vi "SO2 43i Serial Data Recording & DECADEv4.3.vi"() -> ()   [LabVIEW 2014]
uses:
  <vilib>/Instr/_visa.llb/VISA Set IO Buffer Mask.ctl
  <vilib>/Platform/TimedLoop/XDataNode/timing_clust.ctl
  <vilib>/Platform/TimedLoop/XDataNode/nitl_modes.ctl
  <vilib>/Platform/TimedLoop/XDataNode/wakeup.ctl
  C:/Program Files (x86)/National Instruments/LabVIEW 2014/examples/Data Communication/Network Streams/Simple Network Streams/support/Network Stream Command.ctl
  <vilib>/Utility/error.llb/whitespace.ctl
  <vilib>/Instr/_visa.llb/VISA Configure Serial Port (Instr).vi
  <vilib>/Utility/file.llb/Read From Spreadsheet File (string).vi
  <vilib>/Utility/tcp.llb/UDP Multicast Write-Only Open.vi
  <vilib>/platform/TimedLoop/XDataNode/XDataNode.xnode
  <vilib>/Platform/TimedLoop/XDataNode/XDNodeRunTimeDep.lvlib
  <vilib>/ptbypt/NI_PtbyPt.lvlib
panel:
  out "local\ndummy":bool
  out "cal gas cylinder conc":dbl=500.0 format="%.4g"
  out "calcon save to file":bool
  out "ev8 zero interval":i32=600
  out "Auto Zeroing":bool
  out "Simulate MOCCA Conc":dbl
  out "MOCCA window delay time (sec)":i32=30
  out "MOCCA SO2 Limit":i32=800
  out "SO2 Inflight MOCCA Alarm\n(default = OFF)":bool
  out "ev8 user set time":i32=60
  out "Mean Cal Offset":dbl
  out "Mean Cal\n(default = ON)":bool=TRUE
  out "Default file name":string
  out "Stop File Write":bool
  out "error out 4":errorcluster
  out "V6":bool
  out "V8":bool
  out "V9":bool
  out "error out 2":errorcluster
  in  "MFC_2 SLPM set value":dbl
  out "Value Read 2":string
  out "status 2":bool
  out "MFC 2":dbl[](array[numeric])
  in  "VISA resource name 3":refnum<visa-resource-name>="ASRL4::INSTR"
  in  "timeout (10sec) 3":u32=3000
  out "error out 3":errorcluster
  in  "MFC_3 SLPM set value":dbl=2.0
  out "Value Read 3":string
  out "status":bool
  out "MFC 3":dbl[](array[numeric])
  in  "VISA resource name 2":refnum<visa-resource-name>="ASRL5::INSTR"
  in  "timeout (10sec) 2":u32=3000
  out "Data Array UDP":string[](array[string])
  out "Slope":dbl=1.1
  out "Zero":dbl
  out "Simulate TWA Conc":dbl
  out "8hr_TWA_limit":i32=490
  out "10mins_STEL_limit":i32=800
  out "Simulate STEL Conc":dbl
  out "Simulate\nconc":bool
  out "q_size 2":i32
  out "8hr_so2_avg 2":dbl=1.0
  out "10min_so2_avg":dbl=1.0
  out "q_size":i32
  in  "Clear Display\nErrors":bool
  out "Data Processing":bool
  out "Serial Visa Error":errorcluster
  out "SEPTIC TCP Error Out":errorcluster
  out "TCP packet\nSend to SEPTIC":bool
  out "UDP Time Stamp Offset":i32=1
  out "Data Array TCP":string[](array[string])
  out "UDP packet \nstatus":bool
  out "UDP_Out_Error":errorcluster
  out "FISH TCP Error Out":errorcluster
  out "TCP packet\nSend to FISH":bool
  out "TCP Binary Packet":string
  out "Scan from String Error Counter\nfrom process loop":i32
  out "Read Error Counter\nfrom process loop":i32
  in  "milliseconds to wait":u32=330
  in  "ID":string="µ"
  in  "VISA resource name":refnum<visa-resource-name>="ASRL6::INSTR"
  out "Data In Array":string[](array[string])
  out "UDP_ASCII_Out":string
  out "UDP_Pack_num":u32
  out "Flight Number":string
  in  "dummy":string="00"
  out "Data String":string
  out "Internal packet":string[](array[string])
  out "RAW DATA":string
  in  "stop":bool
  out "Time taken history":u32(graph)
  out "Max Acq Time diff":u32
  out "Acq Time":u32
  out "Number of Send & Read Error\nfrom Acquire Loop":i32
  out "Command In":string
  # "SO2_conc"
  # "PMT_Volt"
  # "Lamp_Volt"
  # "Lamp_Intensity_Hz"
  # "Internal_Temp_degC"
  # "Reaction_Chamber_Temp_degC"
  # "Reaction_Chamber_Press_mmHg"
  # "Sample_Flow_litre_per_minute"
  # "Flag"
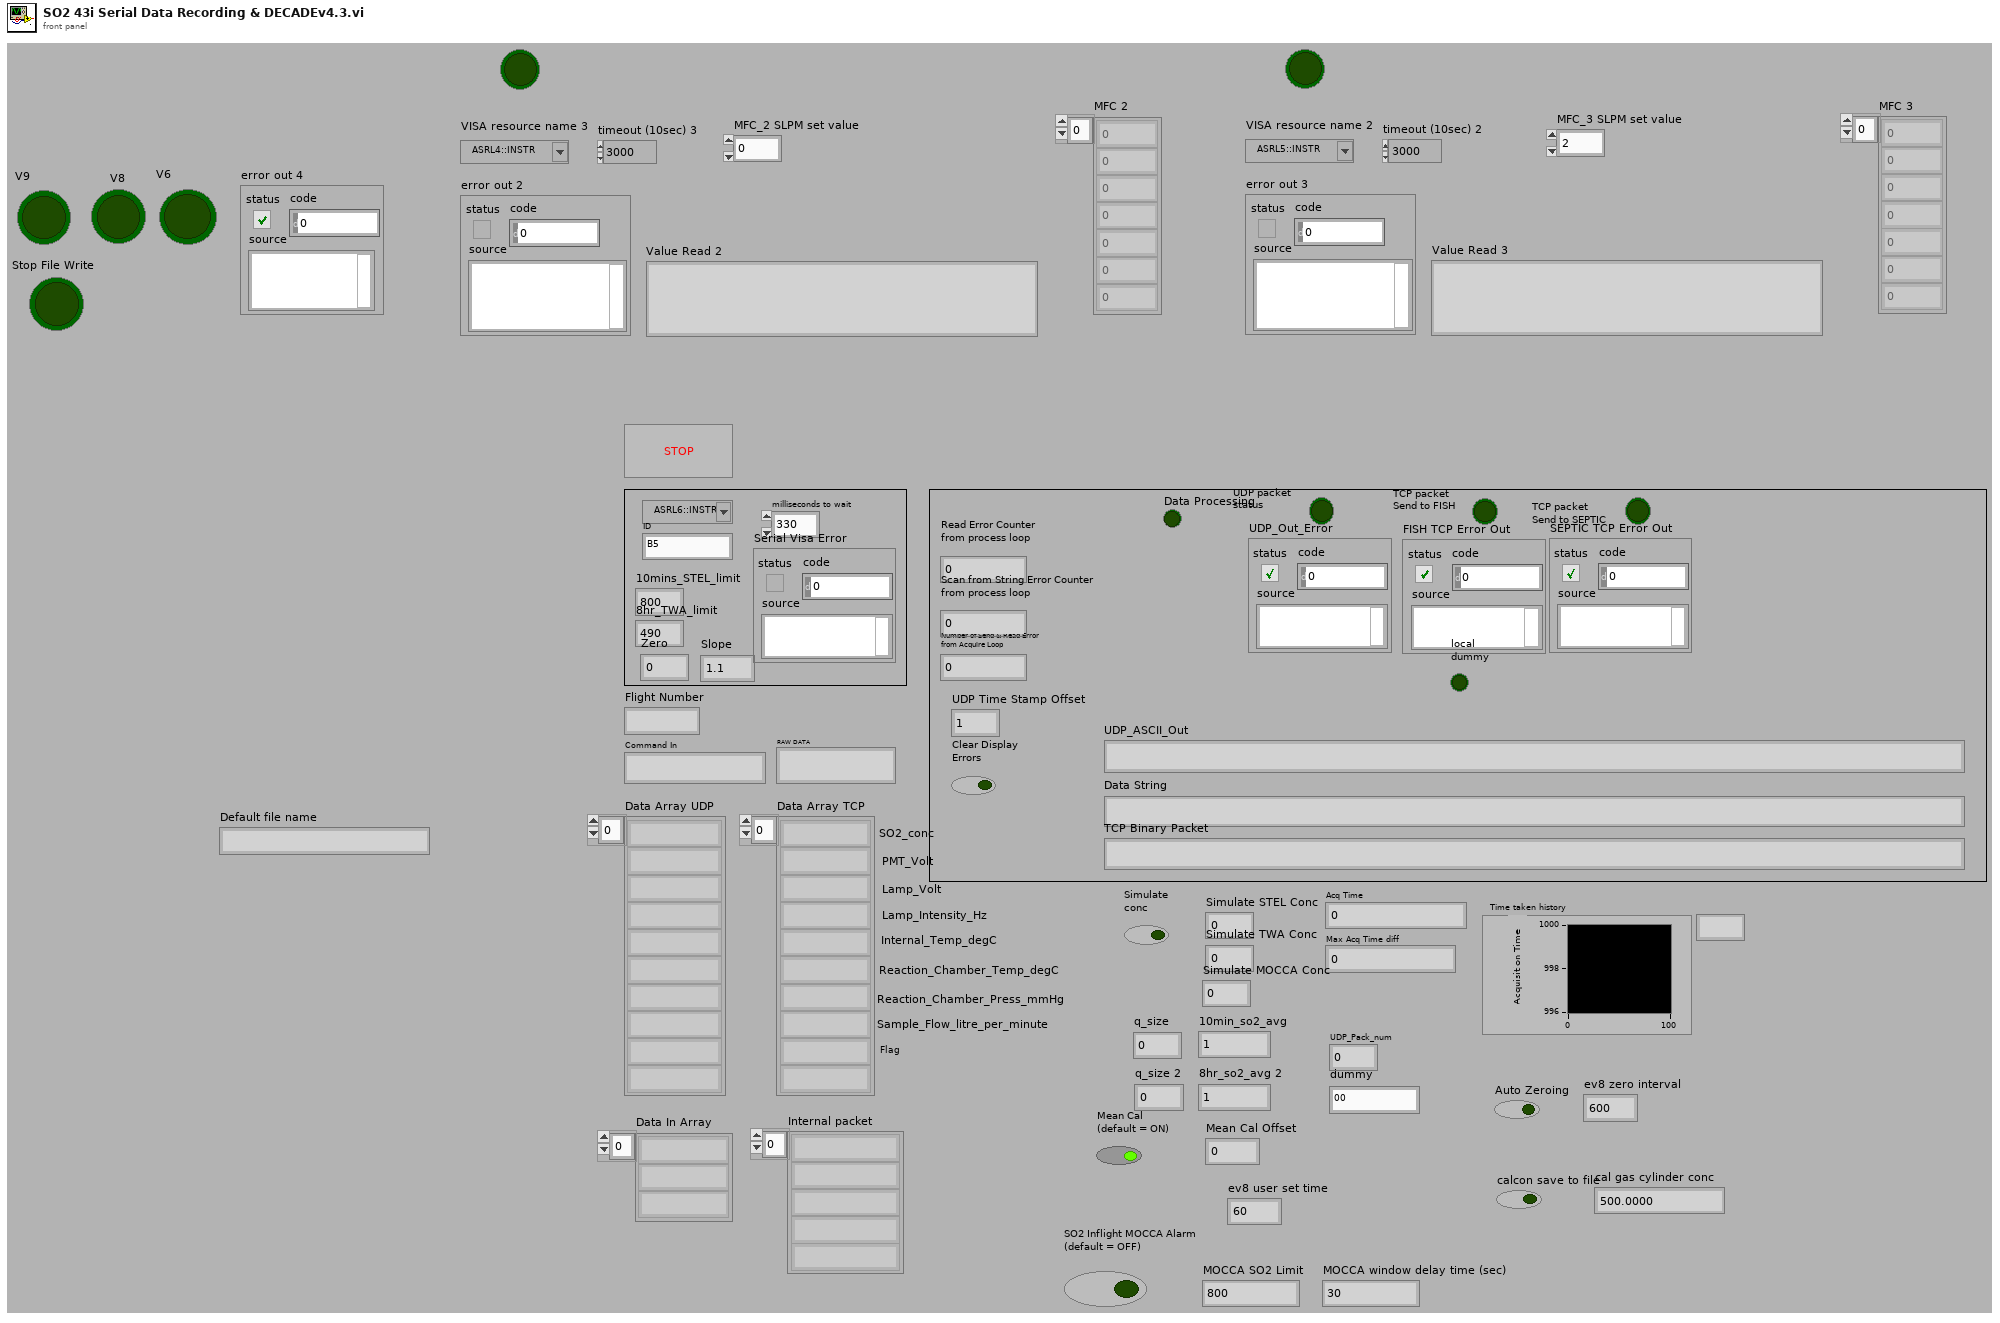
[diagram p1: front panel]
types:
  T1 = typedef "VISA Set IO Buffer Mask.ctl" = u16
  T2 = enum16{"open", "replace", "create", "open or create", "replace or create", "replace or create with confirmation"}
  T3 = typedef "Network Stream Command.ctl" = cluster{"Message":string, "Message Data":variant}
  T4 = typedef "XDNodeRunTimeDep.lvlib/timing_clust.ctl" = cluster{"Expected End [f-1]":u64, "Actual End [f-1]":u64, "Finished Late? [f-1]":bool, "Expected End [i-1]":u64, "Actual End [i-1]":u64, "Finished Late? [i-1]":bool, "Expected Start [i]":u64, "Actual Start [i]":u64, "Expected Start [f]":u64, "Actual Start [f]":u64, "Source Name":string, "Structure Name":string, "Period":i64, "Deadline":i64, "Offset":i64, "Start":i64, "Priority":i32, "Timeout":i32, "Mode":T5, "Wakeup Reason":T6, "Error":errorcluster, "Source Type":string, "Secondary Source Type":string, "Global End Time":u64, "Global Start Time":u64, "Frame Duration":u64, "Iteration Duration":u64, "Assigned CPU":i32, "I/O Scan Engine Mode":u32}
  T5 = typedef "XDNodeRunTimeDep.lvlib/nitl_modes.ctl" = enum32{"No Change", "Process missed periods, maintain original phase", "Discard missed periods, maintain original phase", "Process missed periods, ignore original phase", "Discard missed periods, ignore original phase"}
  T6 = typedef "XDNodeRunTimeDep.lvlib/wakeup.ctl" = enum32{"Normal", "Aborted", "Asynchronous wakeup", "Timing source error", "Timed loop error", "Timeout"}
  T7 = typedef "whitespace.ctl" = u16
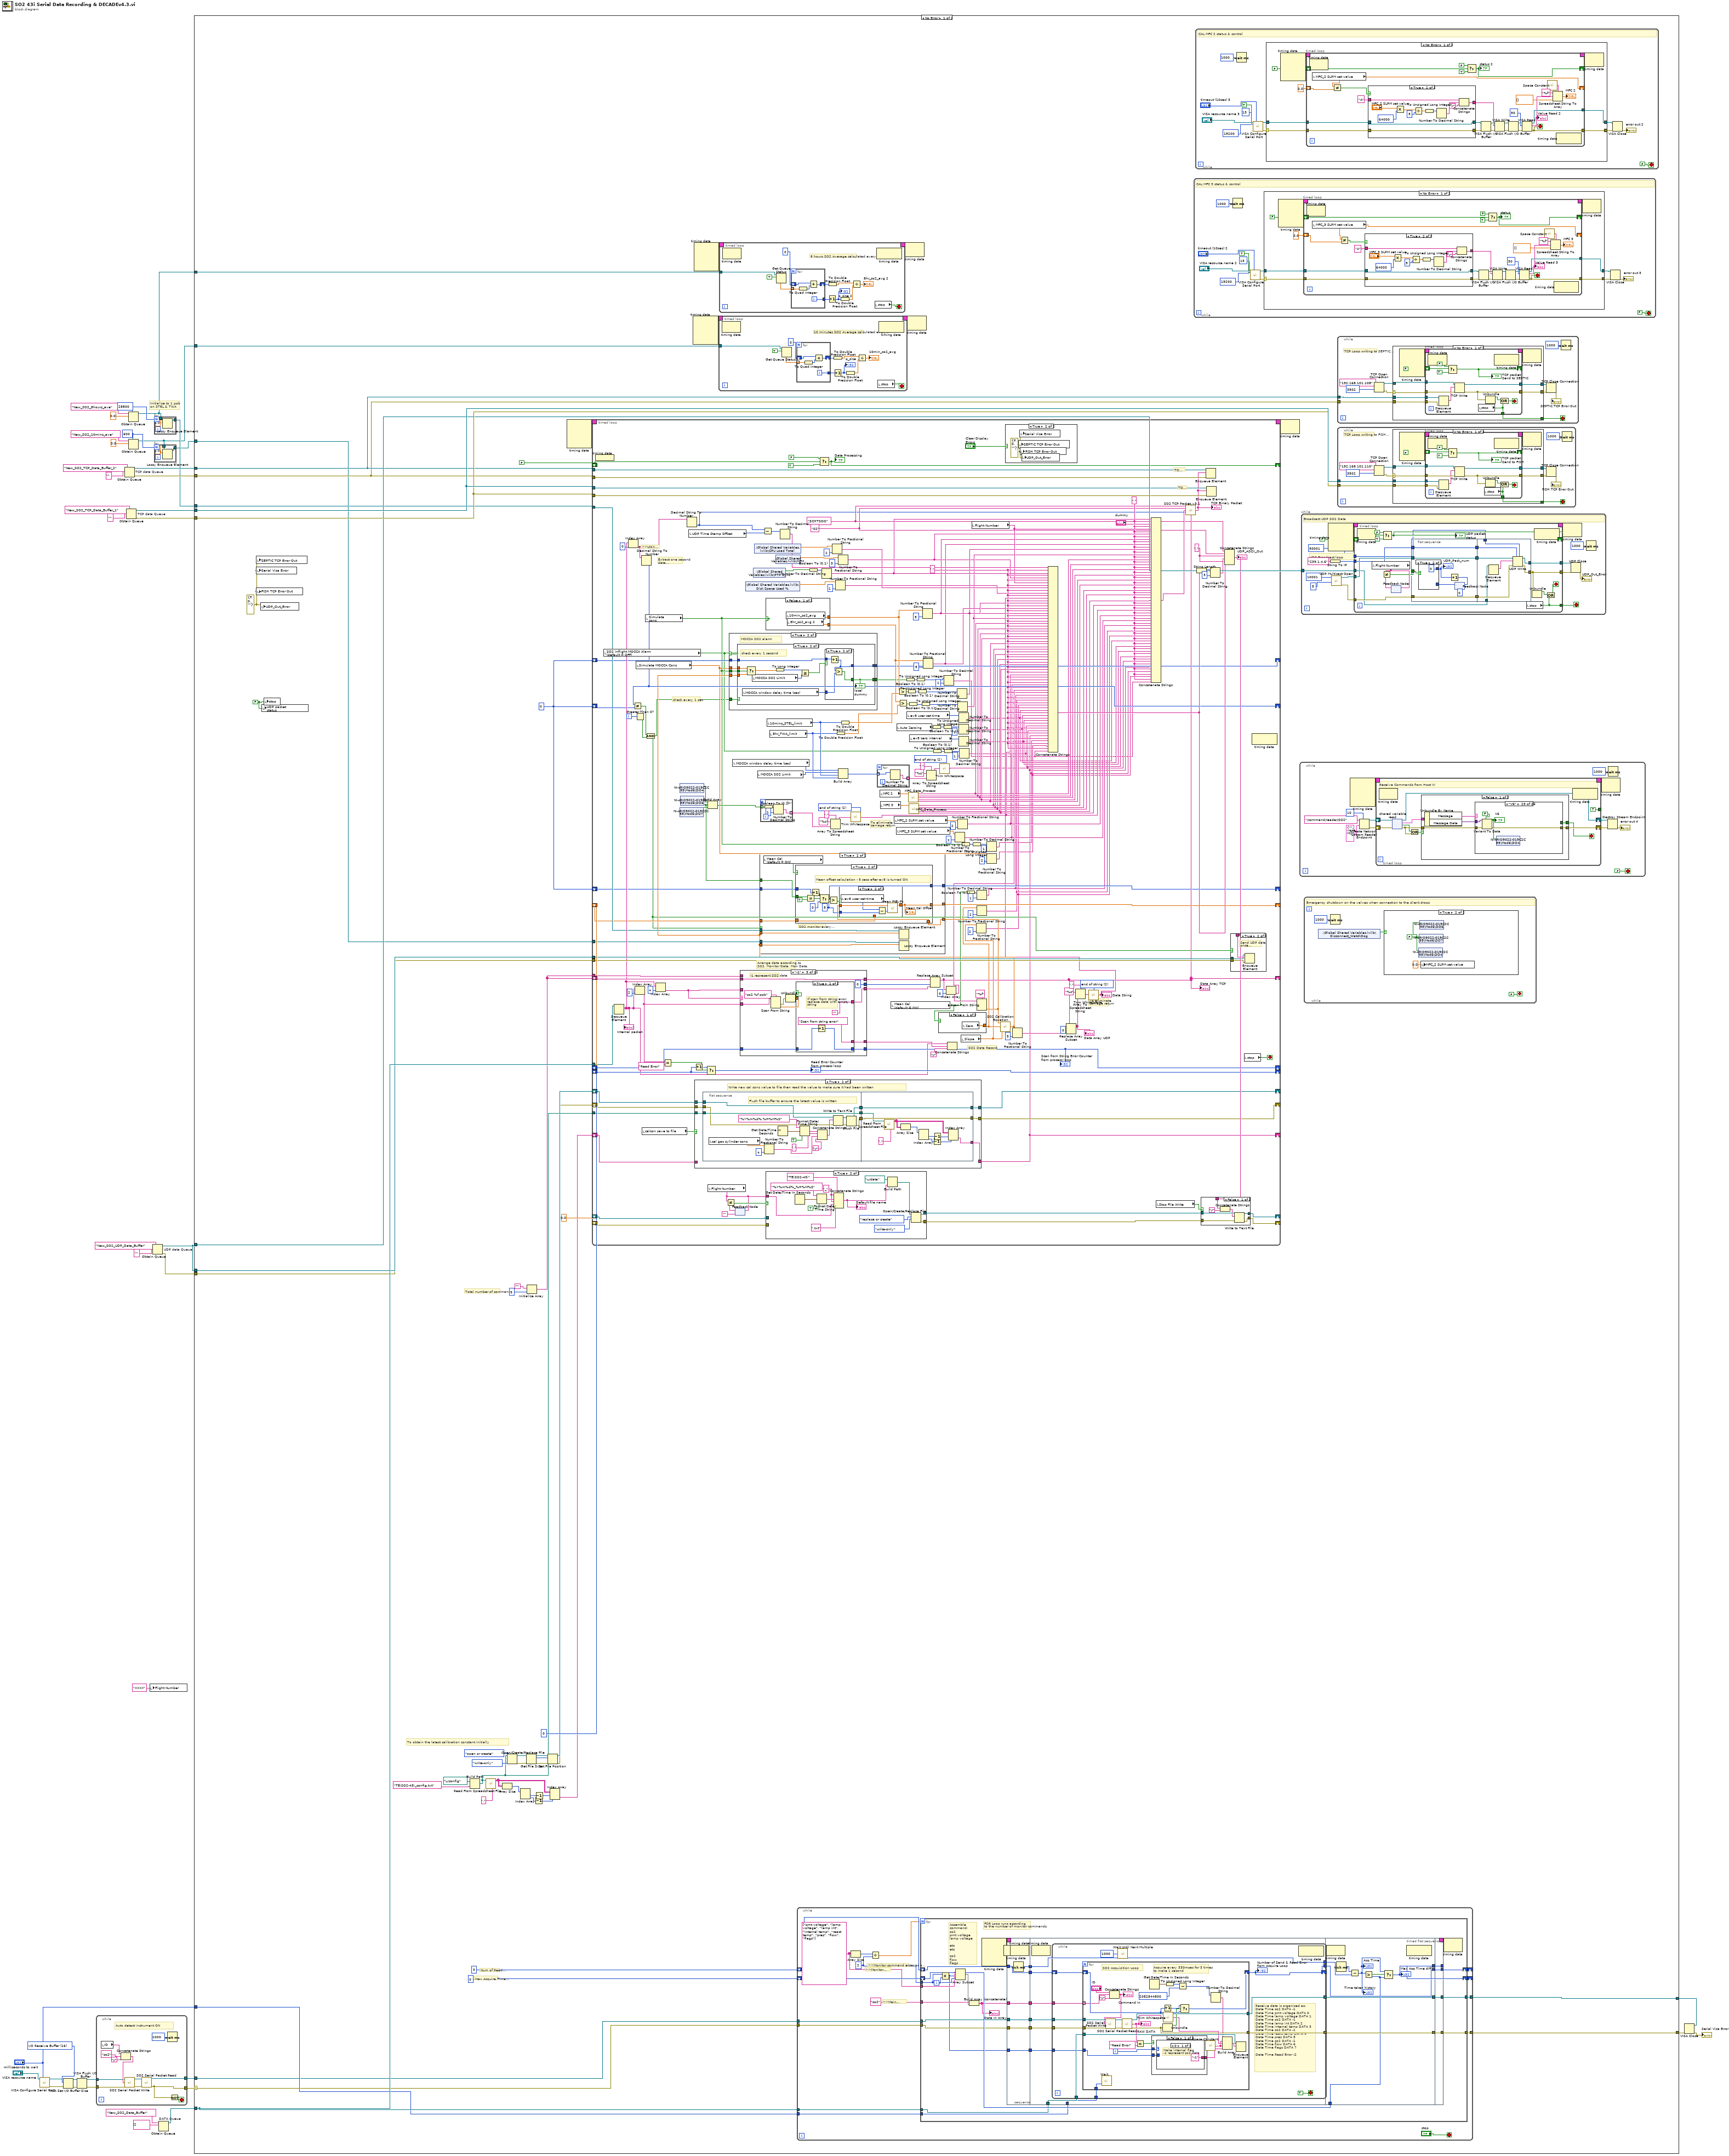
[diagram p0: block diagram]
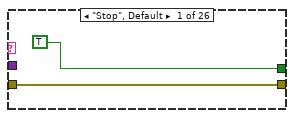
[diagram p3: hidden frame]
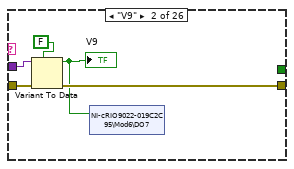
[diagram p4: hidden frame]
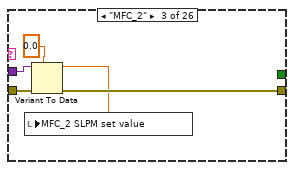
[diagram p5: hidden frame]
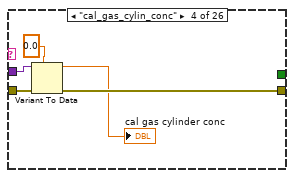
[diagram p6: hidden frame]
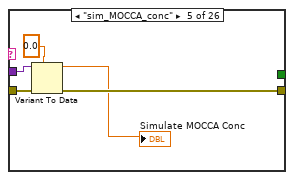
[diagram p7: hidden frame]
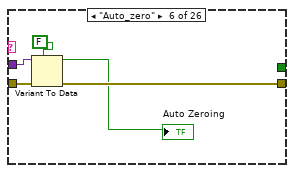
[diagram p8: hidden frame]
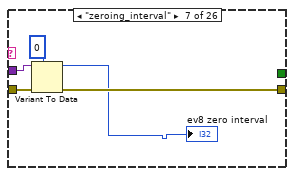
[diagram p9: hidden frame]
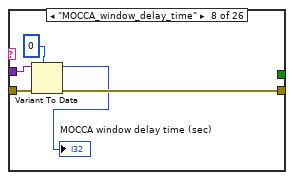
[diagram p10: hidden frame]
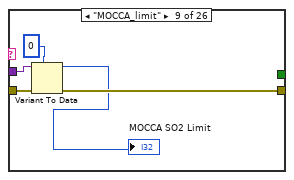
[diagram p11: hidden frame]
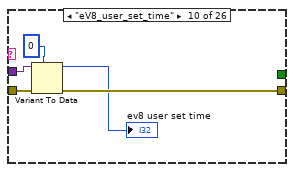
[diagram p12: hidden frame]
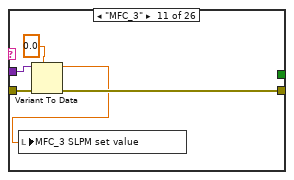
[diagram p13: hidden frame]
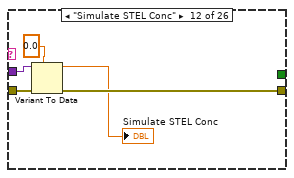
[diagram p14: hidden frame]
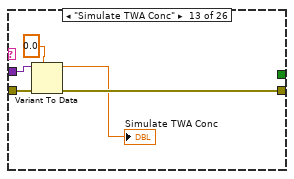
[diagram p15: hidden frame]
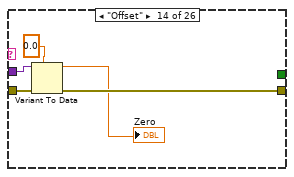
[diagram p16: hidden frame]
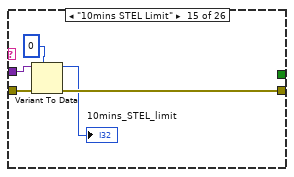
[diagram p17: hidden frame]
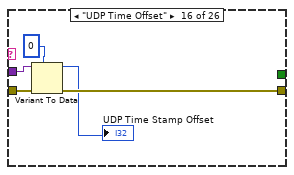
[diagram p18: hidden frame]
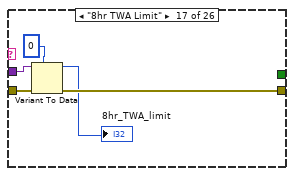
[diagram p19: hidden frame]
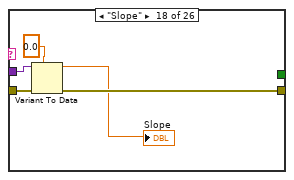
[diagram p20: hidden frame]
diagram:
  w9 = T1 16 items=["I/O Receive Buffer"=16, "I/O Transmit Buffer"=32, "I/O Receive and Transmit Buffer"=48] ("Mask")
  w16 = 28800 ("max queue size (-1, unlimited)")
  w13 = 600 ("max queue size (-1, unlimited)")
  # "Initialise to 1 ppb\non STEL & TWA"
  n1 = call-poly "VISA Configure Serial Port"("VISA resource name"="VISA resource name", "timeout (10sec)"="milliseconds to wait") -> ("VISA resource name out"=w8:refnum<visa-resource-name>, "error out"=w7:errorcluster)  [unwired: 12 in]
  n2 = VISA Set I/O Buffer Size(VISA resource name=w8, mask (16)=w9, error in (no error)=w7) -> (VISA resource name out=w2:refnum<visa-resource-name>, error out=w10:errorcluster)  [unwired: 1 in]
  n3 = VISA Flush I/O Buffer(VISA resource name=w2, error in (no error)=w10) -> (VISA resource name out=w6:refnum<visa-resource-name>, error out=w5:errorcluster)  [unwired: 1 in]
  n4 = while {
    tunnel: w6 -> [w45]
    tunnel: w5 -> [w44]
    tunnel: [w43] -> w4
    tunnel: [w42] -> w3
    stop <- w41 stop-if-true
    # "Auto detect instrument ON"
    n5 = local read "ID"() -> (w46:string)
    n6 = Concatenate Strings(w46, "so2" ("string"), "\r") -> (w49:string)
    n7 = call "SO2 Serial Packet Write.vi"("VISA resource name In"=w45, "Data in"=w49, "error in (no error)"=w44) -> ("VISA resource name Out"=w51:refnum<visa-resource-name>, "error out"=w50:errorcluster)  [unwired: 11 in]
    n8 = call "SO2 Serial Packet Read.vi"("VISA resource In"=w51, "error in"=w50) -> ("VISA resource Out"=w42:refnum<visa-resource-name>, "error out"=w43:errorcluster)  [unwired: 11 in, 1 out]
    n9 = Wait (ms)(milliseconds to wait=u32 1000) -> ()  [unwired: 1 out]
    n10 = Not(x=w43) -> (.not. x?=w41:bool)
  }
  n11 = Obtain Queue "TCP data Queue"(name (unnamed)="New_SO2_TCP_Data_Buffer_2", element data type="") -> (queue out=w23:refnum<queue>, error out=w22:errorcluster)  [unwired: 3 in, 1 out]
  n12 = Obtain Queue "TCP data Queue"(name (unnamed)="New_SO2_TCP_Data_Buffer_1", element data type="") -> (queue out=w31:refnum<queue>, error out=w30:errorcluster)  [unwired: 3 in, 1 out]
  n13 = Obtain Queue(max queue size (-1, unlimited)=w16, name (unnamed)="New_SO2_8hours_ave", element data type=0.0 ("index")) -> (queue out=w15:refnum<queue>)  [unwired: 2 in, 2 out]
  n14 = Obtain Queue(max queue size (-1, unlimited)=w13, name (unnamed)="New_SO2_10mins_ave", element data type=0.0 ("index")) -> (queue out=w12:refnum<queue>)  [unwired: 2 in, 2 out]
  n15 = local write "Flight Number"("XXXX" ("Flight Number")) -> ()
  n16 = Obtain Queue "UDP data Queue"(name (unnamed)="New_SO2_UDP_Data_Buffer", element data type="") -> (queue out=w26:refnum<queue>, error out=w27:errorcluster)  [unwired: 3 in, 1 out]
  n17 = for {
    N: w16 -> [_]
    tunnel: w15 -> [w55]
    tunnel: [w54] -> w14
    n18 = Lossy Enqueue Element(queue=w55, element=1.0) -> (queue out=w54:refnum<queue>)  [unwired: 1 in, 3 out]
  }
  n19 = for {
    N: w13 -> [_]
    tunnel: [w58] -> w11
    tunnel: w12 -> [w56]
    n20 = Lossy Enqueue Element(queue=w56, element=1.0) -> (queue out=w58:refnum<queue>)  [unwired: 1 in, 3 out]
  }
  n21 = Obtain Queue "DATA Queue"(name (unnamed)="New_SO2_Data_Buffer", element data type=string[] []) -> (queue out=w38:refnum<queue>)  [unwired: 3 in, 2 out]
  n22 = case shown="No Error" w4 {
    selector: w4 -> [w81 w1296]
    tunnel: [w112 w1296] -> w35
    tunnel: [w111 w1295] -> w36
    tunnel: w38 -> [w108 _]
    tunnel: w3 -> [w82 w1295]
    tunnel: w31 -> [w100 _]
    tunnel: w30 -> [w99 _]
    tunnel: w26 -> [w98 _]
    tunnel: w27 -> [w97 _]
    tunnel: w26 -> [w96 _]
    tunnel: w23 -> [w95 _]
    tunnel: w22 -> [w94 _]
    tunnel: "milliseconds to wait" -> [w93 _]
    tunnel: w12 -> [w90 _]
    tunnel: w15 -> [w89 _]
    tunnel: w11 -> [w88 _]
    tunnel: w14 -> [w87 _]
    frame No Error {
      w79 = 0
      w91 = errorcluster {"status"=FALSE, "code"=0, "source"=""} ("UDP Error Out")
      w102 = 0
      w101 = FALSE ("stop")
      # "To obtain the latest calibration constant initially"
      # "Max Acquire Time Diff"
      # "Num of Read Error"
      # "Total number of commands"
      n23 = local write "SEPTIC TCP Error Out"(w91) -> ()
      n24 = local write "Serial Visa Error"(w91) -> ()
      n25 = local write "FISH TCP Error Out"(w91) -> ()
      n26 = local write "UDP_Out_Error"(w91) -> ()
      n27 = local write "UDP packet \nstatus"(w101) -> ()
      n28 = local write "stop"(w101) -> ()
      n29 = Build Path(base path=path "u:/config", name or relative path="TEiSO2-43i_config.txt" ("string")) -> (appended path=w61:path)
      n30 = call-poly <vilib>:"Read From Spreadsheet File.vi"("delimiter (\\t)"="," ("delimiter (\\t)"), "file path (dialog if empty)"=w61) -> ("all rows"=w70:string[][])  [unwired: 5 in, 4 out]
      n31 = Array Size(array=w70) -> (size(s)=w71:i32[])
      n32 = Open/Create/Replace File(file path (use dialog)=w61, operation (0:open)=T2."open or create", access (0:read/write)=enum16{"read/write", "read-only", "write-only"}."write-only") -> (refnum out=w63:refnum<file>, error out=w64:errorcluster)  [unwired: 3 in, 1 out]
      n33 = Index Array(array=w71) -> (element #1=w75:i32, element #2=w73:i32)  [unwired: 2 in]
      n34 = Get File Size(file=w63, error in=w64) -> (refnum out=w65:refnum<file>, size (in bytes)=w67:i64, 0:w66:errorcluster)
      n35 = Initialize Array("", 9) -> (w103:string[])
      n36 = Decrement(x=w73) -> (x-1=w72:i32)
      n37 = Decrement(x=w75) -> (x-1=w74:i32)
      n38 = Set File Position(offset (in bytes) (0)=w67, refnum=w65, error in=w66) -> (refnum out=w60:refnum<file>, error out=w59:errorcluster)  [unwired: 1 in]
      n39 = Index Array(array=w70, index (row)=w74, index (col)=w72) -> (element=w69:string)
      n40 = node-c288() -> (w110:T4)  [unwired: 4 in]
      n41 = timed-loop {
        timing: w110 -> [_]
        timing-out: [_] -> w109
        tunnel: w108 -> [w945]
        shift-right: [w877] -> _
        shift-left: w103 -> [w935]
        shift-right: [w926] -> _
        shift-left: w102 -> [w923]
        tunnel: w103 -> [w925]
        shift-right: [w921] -> _
        shift-left: w102 -> [w922]
        tunnel: w100 -> [w919]
        tunnel: w99 -> [w918]
        tunnel: w98 -> [w917]
        tunnel: w97 -> [w916]
        shift-right: [w908] -> _
        shift-left: w79 -> [w911]
        tunnel: w95 -> [w907]
        tunnel: w94 -> [w906]
        shift-right: [w899] -> _
        shift-left: FALSE -> [w902]
        tunnel: w88 -> [w896]
        tunnel: w87 -> [w895]
        shift-right: [w864] -> _
        shift-left: _ -> [w866]
        shift-right: [w863] -> _
        shift-left: _ -> [w865]
        shift-right: [w833] -> _
        shift-left: w79 -> [w835]
        shift-right: [w831] -> _
        shift-left: 0.0 -> [w832]
        shift-right: [w821] -> _
        shift-left: w79 -> [w822]
        tunnel: w61 -> [w798]
        shift-right: [w752] -> _
        shift-left: w69 -> [w797]
        shift-right: [w788] -> _
        shift-left: w60 -> [w789]
        shift-right: [w786] -> _
        shift-left: w59 -> [w787]
        i -> [w909]
        stop <- w943 stop-if-true
        w749 = ","
        (unwired) i16 1 ("width (-)")
        (unwired) T7 2 items=["both", "start of string", "end of string"] ("location (both)")
        w841 = T7 2 items=["both", "start of string", "end of string"] ("location (both)")
        w931 = T7 2 items=["both", "start of string", "end of string"] ("location (both)")
        w791 = ","
        w745 = "02"
        w937 = ","
        w746 = "$CHTSOO"
        # "check every 1 sec"
        # "To eliminate\ncarriage return"
        # "TO SEPTIC"
        # "TO FISH"
        # "Extract one second data\nfor UDP sending"
        # "Arrange data according to\nSO2, Monitor Data, Mon Data,"
        # "To eliminate\ncarriage return"
        # ">>UNIX TIME>>"
        # "SO2 Data Record"
        n42 = node-c288() -> ()  [unwired: 1 in]
        n43 = local read "SO2 Inflight MOCCA Alarm\n(default = OFF)"() -> (w784:bool)
        n44 = Dequeue Element(queue=w945) -> (element=w914:string[])  [unwired: 2 in, 3 out]
        "Internal packet" <- w914
        n45 = Index Array(array=w914, index=0) -> (element=w913:string)
        n46 = Index Array(array=w914, index=2) -> (element=w929:string)
        n47 = Greater Than 0?(x=w909) -> (x > 0?=w912:bool)
        n48 = local read "Simulate MOCCA Conc"() -> (w792:dbl)
        n49 = Decimal String To Number(string=w913) -> (number=w908:i32)  [unwired: 2 in, 1 out]
        n50 = Not Equal?(x=w908, y=w911) -> (x != y?=w910:bool)
        n51 = local read "calcon save to file"() -> (w785:bool)
        n52 = local read "Simulate\nconc"() -> (w794:bool)
        n53 = Compound Arithmetic op=AND(w910, w912) -> (w783:bool)
        n54 = Index Array(array=w914, index=4) -> (element=w898:string)
        n55 = Equal?(x=w929, y="Read Error") -> (x = y?=w927:bool)
        n56 = shared-variable "NI-cRIO9022-019C2C95\\Mod6\\DO7"() -> (w849:bool)  [unwired: 1 in, 1 out]
        n57 = shared-variable "NI-cRIO9022-019C2C95\\Mod6\\DO4"() -> (w850:bool)  [unwired: 1 in, 1 out]
        n58 = shared-variable "NI-cRIO9022-019C2C95\\Mod6\\DO6"() -> (w836:bool)  [unwired: 1 in, 1 out]
        n59 = Decimal String To Number(string=w913) -> (number=w744:i32)  [unwired: 2 in, 1 out]
        n60 = local read "UDP Time Stamp Offset"() -> (w840:i32)
        n61 = Increment(x=w923) -> (x+1=w924:i32)
        n62 = case shown="True" w785 {
          tunnel: w798 -> [_ w957]
          tunnel: [w946 w955] -> w786
          tunnel: w797 -> [w948 _]
          tunnel: [w948 w954] -> w752
          tunnel: w789 -> [w947 w952]
          tunnel: [w947 w950] -> w788
          tunnel: w787 -> [w946 w949]
          frame False {
          }
          frame True {
            # "Write new cal conc value to file then read the value to make sure it had been written"
            n63 = flat-sequence {
              tunnel: w957 -> [w965]
              tunnel: [w960] -> w956
              tunnel: [w965] -> w953
              tunnel: w952 -> [w964]
              tunnel: [w959] -> w951
              tunnel: w949 -> [w963]
              tunnel: w956 -> [w978]
              tunnel: [w978] -> w955
              tunnel: [w977] -> w954
              tunnel: w953 -> [w976]
              tunnel: w951 -> [w975]
              tunnel: [w975] -> w950
              frame #0 {
                # "Flush file buffer to ensure the latest value is written"
                n64 = local read "cal gas cylinder conc"() -> (w958:dbl)
                n65 = Number To Fractional String(number=w958, precision (6)=i16 4) -> (F-format string=w966:string)  [unwired: 2 in]
                n66 = Get Date/Time In Seconds() -> (seconds since 1Jan1904=w973:timestamp)
                n67 = Format Date/Time String(time format string (%c)="%Y%m%d%,%H%M%S", seconds (now)=w973, UTC format=TRUE) -> (date/time string=w970:string)
                n68 = Concatenate Strings(w970, "," ("string"), w966, "\r") -> (w968:string)
                n69 = Write to Text File(file (use dialog)=w964, text=w968, error in=w963) -> (refnum out=w961:refnum<file>, error out=w962:errorcluster)  [unwired: 1 in, 1 out]
                n70 = Flush File(refnum=w961, error in=w962) -> (refnum out=w959:refnum<file>, error out=w960:errorcluster)
              }
              frame #1 {
                n71 = call-poly <vilib>:"Read From Spreadsheet File.vi"("delimiter (\\t)"="," ("delimiter (\\t)"), "file path (dialog if empty)"=w976) -> ("all rows"=w979:string[][])  [unwired: 5 in, 4 out]
                n72 = Array Size(array=w979) -> (size(s)=w980:i32[])
                n73 = Index Array(array=w980) -> (element #1=w984:i32, element #2=w982:i32)  [unwired: 2 in]
                n74 = Decrement(x=w982) -> (x-1=w981:i32)
                n75 = Decrement(x=w984) -> (x-1=w983:i32)
                n76 = Index Array(array=w979, index (row)=w983, index (col)=w981) -> (element=w977:string)
              }
            }
          }
        }
        n77 = Select(t=w924, s=w927, f=w923) -> (s? t:f=w926:i32)
        "Read Error Counter\nfrom process loop" <- w926
        n78 = Build Array(w850, w836, w849) -> (w854:bool[])
        n79 = local read "Flight Number"() -> (w867:string)
        n80 = local read "MOCCA window delay time (sec)"() -> (w803:i32)
        n81 = feedback #1("" ("Flight Number")) -> (w872:string)
        n82 = Not Equal?(x=w867, y=w872) -> (x != y?=w870:bool)
        n83 = feedback-in #1(w867) -> ()
        n84 = case shown="\"-1\"" w898 {
          tunnel: w898 -> [w1094 _ _ w1130 w1151 w1172 w1194 w1216 w1238 w1260 w1282]
          tunnel: w935 -> [w1095 _ w1109 w1131 w1152 w1173 w1195 w1217 w1239 w1261 w1283]
          tunnel: w929 -> [_ _ w1106 w1126 w1147 w1169 w1191 w1213 w1235 w1257 w1279]
          tunnel: [w1095 w1098 w1109 w1131 w1152 w1173 w1195 w1217 w1239 w1261 w1283] -> w882
          tunnel: [w1092 _ 0 ("index") w1128 w1149 w1170 w1192 w1214 w1236 w1258 w1280] -> w881
          tunnel: [_ _ w1105 w1125 w1146 w1168 w1190 w1212 w1234 w1256 w1274] -> w934
          tunnel: w925 -> [_ w1098 _ _ _ _ _ _ _ _ _]
          tunnel: w922 -> [w1090 w1097 w1102 w1122 w1143 w1163 w1186 w1207 w1230 w1251 w1273]
          tunnel: [w1090 w1097 w1101 w1121 w1142 w1162 w1185 w1206 w1229 w1250 w1272] -> w921
          tunnel: ["Internal False Flag Detected" "" w1100 w1120 w1141 w1161 w1184 w1205 w1228 w1249 w1271] -> w920
          frame "False", Default {
            n85 = Decimal String To Number(string=w1094) -> (number=w1091:i32)  [unwired: 2 in, 1 out]
            n86 = Add(x=w1091, y=1) -> (x+y=w1092:i32)
          }
          frame "-2" {
            # "Read Error Detected\nMake all data as a space"
          }
          frame "-1" {
            # "-1 represent SO2 data"
            n87 = Scan From String(format string="so2 %f ppb", input string=w1106) -> (error out=w1104:errorcluster, output 1=w1099:dbl)  [unwired: 3 in, 2 out]
            n88 = Unbundle(w1104) -> ("status"=w1103:bool)  [unwired: 2 out]
            n89 = case shown="True" w1103 {
              tunnel: w1099 -> [w1110 _]
              tunnel: [w1114 ""] -> w1105
              tunnel: w1102 -> [w1113 w1118]
              tunnel: [w1113 w1117] -> w1101
              tunnel: ["" "Scan from string error"] -> w1100
              frame False {
                # "Extract the concentration\nvalue & fixed format"
                n90 = Number To Fractional String(number=w1110, precision (6)=i16 5) -> (F-format string=w1114:string)  [unwired: 2 in]
              }
              frame True {
                # "If scan from string error,\nreplace data with empty\nstring"
                n91 = Increment(x=w1118) -> (x+1=w1117:i32)
              }
            }
          }
          frame "0" {
            # "0 represents pmt voltage -0510 volts"
            n92 = Scan From String(format string="pmt voltage %d", input string=w1126) -> (error out=w1124:errorcluster, output 1=w1119:i32)  [unwired: 3 in, 2 out]
            n93 = Decimal String To Number(string=w1130) -> (number=w1129:i32)  [unwired: 2 in, 1 out]
            n94 = Unbundle(w1124) -> ("status"=w1123:bool)  [unwired: 2 out]
            n95 = case shown="False" w1123 {
              tunnel: w1119 -> [w1135 _]
              tunnel: [w1132 w1136] -> w1125
              tunnel: w1122 -> [w1134 w1139]
              tunnel: [w1134 w1138] -> w1121
              tunnel: ["" "Scan from string error"] -> w1120
              tunnel: [w1132 w1136] -> _
              frame False {
                # "Extract the actual value\n& fixed format"
                n96 = Number To Decimal String(number=w1135) -> (decimal integer string=w1132:string)  [unwired: 1 in]
              }
              frame True {
                w1136 = ""
                # "If scan from string error,\nreplace data with empty\nstring"
                n97 = Increment(x=w1139) -> (x+1=w1138:i32)
              }
            }
            n98 = Increment(x=w1129) -> (x+1=w1128:i32)
          }
          frame "1" {
            # "1 represents lamp voltage; lamp voltage 810 volts"
            n99 = Scan From String(format string="lamp voltage %d", input string=w1147) -> (error out=w1145:errorcluster, output 1=w1140:i32)  [unwired: 3 in, 2 out]
            n100 = Decimal String To Number(string=w1151) -> (number=w1150:i32)  [unwired: 2 in, 1 out]
            n101 = Unbundle(w1145) -> ("status"=w1144:bool)  [unwired: 2 out]
            n102 = case shown="True" w1144 {
              tunnel: w1140 -> [w1156 _]
              tunnel: [w1153 w1157] -> w1146
              tunnel: w1143 -> [w1155 w1160]
              tunnel: [w1155 w1159] -> w1142
              tunnel: ["" "Scan from string error"] -> w1141
              tunnel: [w1153 w1157] -> _
              frame False {
                # "Extract the actual value\n& fixed format"
                n103 = Number To Decimal String(number=w1156) -> (decimal integer string=w1153:string)  [unwired: 1 in]
              }
              frame True {
                w1157 = ""
                # "If scan from string error,\nreplace data with empty\nstring"
                n104 = Increment(x=w1160) -> (x+1=w1159:i32)
              }
            }
            n105 = Increment(x=w1150) -> (x+1=w1149:i32)
          }
          frame "2" {
            # "2 represents lamp intensity; lamp int 35867 Hz"
            n106 = Scan From String(format string="lamp int %d", input string=w1169) -> (error out=w1165:errorcluster, output 1=w1166:i32)  [unwired: 3 in, 2 out]
            n107 = Decimal String To Number(string=w1172) -> (number=w1171:i32)  [unwired: 2 in, 1 out]
            n108 = Unbundle(w1165) -> ("status"=w1164:bool)  [unwired: 2 out]
            n109 = case shown="True" w1164 {
              tunnel: [w1174 w1179] -> w1168
              tunnel: w1166 -> [w1178 _]
              tunnel: w1163 -> [w1177 w1182]
              tunnel: [w1177 w1181] -> w1162
              tunnel: ["" "Scan from string error"] -> w1161
              tunnel: [w1174 w1179] -> _
              frame False {
                # "Extract the actual value\n& fixed format"
                n110 = Number To Fractional String(number=w1178, precision (6)=i16 0) -> (F-format string=w1174:string)  [unwired: 2 in]
              }
              frame True {
                w1179 = ""
                # "If scan from string error,\nreplace data with empty\nstring"
                n111 = Increment(x=w1182) -> (x+1=w1181:i32)
              }
            }
            n112 = Increment(x=w1171) -> (x+1=w1170:i32)
          }
          frame "3" {
            # "3 represents internal temp; internal temp 027.2 deg C, actual 027.2"
            n113 = Scan From String(format string="%[^,], %s %f", input string=w1191) -> (error out=w1188:errorcluster, output 3=w1183:dbl)  [unwired: 7 in, 2 out]
            n114 = Decimal String To Number(string=w1194) -> (number=w1193:i32)  [unwired: 2 in, 1 out]
            n115 = Unbundle(w1188) -> ("status"=w1187:bool)  [unwired: 2 out]
            n116 = case shown="True" w1187 {
              tunnel: [w1196 w1201] -> w1190
              tunnel: w1183 -> [w1200 _]
              tunnel: w1186 -> [w1199 w1204]
              tunnel: [w1199 w1203] -> w1185
              tunnel: ["" "Scan from string error"] -> w1184
              tunnel: [w1196 w1201] -> _
              frame False {
                # "Extract the actual value\n& fixed format"
                n117 = Number To Fractional String(number=w1200, precision (6)=i16 1) -> (F-format string=w1196:string)  [unwired: 2 in]
              }
              frame True {
                w1201 = ""
                # "If scan from string error,\nreplace data with empty\nstring"
                n118 = Increment(x=w1204) -> (x+1=w1203:i32)
              }
            }
            n119 = Increment(x=w1193) -> (x+1=w1192:i32)
          }
          frame "4" {
            # "4 represents react temp; react temp 045.2 deg C"
            n120 = Scan From String(format string="react temp %f deg C", input string=w1213) -> (error out=w1209:errorcluster, output 1=w1210:dbl)  [unwired: 3 in, 2 out]
            n121 = Decimal String To Number(string=w1216) -> (number=w1215:i32)  [unwired: 2 in, 1 out]
            n122 = Unbundle(w1209) -> ("status"=w1208:bool)  [unwired: 2 out]
            n123 = case shown="False" w1208 {
              tunnel: [w1218 w1223] -> w1212
              tunnel: w1210 -> [w1222 _]
              tunnel: w1207 -> [w1221 w1226]
              tunnel: [w1221 w1225] -> w1206
              tunnel: ["" "Scan from string error"] -> w1205
              tunnel: [w1218 w1223] -> _
              frame False {
                # "Extract the actual value\n& fixed format"
                n124 = Number To Fractional String(number=w1222, precision (6)=i16 1) -> (F-format string=w1218:string)  [unwired: 2 in]
              }
              frame True {
                w1223 = ""
                # "If scan from string error,\nreplace data with empty\nstring"
                n125 = Increment(x=w1226) -> (x+1=w1225:i32)
              }
            }
            n126 = Increment(x=w1215) -> (x+1=w1214:i32)
          }
          frame "5" {
            # "5 represents chamber pressure; pres 760.0 mm Hg, actual 753.4"
            n127 = Scan From String(format string="%[^,], %s %f", input string=w1235) -> (error out=w1232:errorcluster, output 3=w1227:dbl)  [unwired: 7 in, 2 out]
            n128 = Decimal String To Number(string=w1238) -> (number=w1237:i32)  [unwired: 2 in, 1 out]
            n129 = Unbundle(w1232) -> ("status"=w1231:bool)  [unwired: 2 out]
            n130 = case shown="False" w1231 {
              tunnel: [w1240 w1245] -> w1234
              tunnel: w1227 -> [w1244 _]
              tunnel: w1230 -> [w1243 w1248]
              tunnel: [w1243 w1247] -> w1229
              tunnel: ["" "Scan from string error"] -> w1228
              tunnel: [w1240 w1245] -> _
              frame False {
                # "Extract the actual value\n& fixed format"
                n131 = Number To Fractional String(number=w1244, precision (6)=i16 1) -> (F-format string=w1240:string)  [unwired: 2 in]
              }
              frame True {
                w1245 = ""
                # "If scan from string error,\nreplace data with empty\nstring"
                n132 = Increment(x=w1248) -> (x+1=w1247:i32)
              }
            }
            n133 = Increment(x=w1237) -> (x+1=w1236:i32)
          }
          frame "6" {
            # "6 represents flow data; flow 0.503 l/m"
            n134 = Scan From String(format string="flow %f l/m", input string=w1257) -> (error out=w1253:errorcluster, output 1=w1254:dbl)  [unwired: 3 in, 2 out]
            n135 = Decimal String To Number(string=w1260) -> (number=w1259:i32)  [unwired: 2 in, 1 out]
            n136 = Unbundle(w1253) -> ("status"=w1252:bool)  [unwired: 2 out]
            n137 = case shown="True" w1252 {
              tunnel: [w1266 ""] -> w1256
              tunnel: w1254 -> [w1265 _]
              tunnel: w1251 -> [w1264 w1269]
              tunnel: [w1264 w1268] -> w1250
              tunnel: ["" "Scan from string error"] -> w1249
              frame False {
                # "Extract the actual value\n& fixed format"
                n138 = Number To Fractional String(number=w1265, precision (6)=i16 3) -> (F-format string=w1266:string)  [unwired: 2 in]
              }
              frame True {
                # "If scan from string error,\nreplace data with empty\nstring"
                n139 = Increment(x=w1269) -> (x+1=w1268:i32)
              }
            }
            n140 = Increment(x=w1259) -> (x+1=w1258:i32)
          }
          frame "7" {
            # "7 represents flags data; flags 1c100000"
            n141 = Scan From String(format string="flags %s", input string=w1279) -> (error out=w1277:errorcluster, output 1=w1275:string)  [unwired: 3 in, 2 out]
            n142 = Decimal String To Number(string=w1282) -> (number=w1281:i32)  [unwired: 2 in, 1 out]
            n143 = Unbundle(w1277) -> ("status"=w1276:bool)  [unwired: 2 out]
            n144 = case shown="False" w1276 {
              tunnel: w1275 -> [w1286 _]
              tunnel: [w1286 ""] -> w1274
              tunnel: w1273 -> [w1285 w1289]
              tunnel: [w1285 w1288] -> w1272
              tunnel: ["" "Scan from string error"] -> w1271
              frame False {
                # "Extract the actual value\n& fixed format"
              }
              frame True {
                # "If scan from string error,\nreplace data with empty\nstring"
                n145 = Increment(x=w1289) -> (x+1=w1288:i32)
              }
            }
            n146 = Increment(x=w1281) -> (x+1=w1280:i32)
          }
        }
        "Scan from String Error Counter\nfrom process loop" <- w921
        n147 = shared-variable ".\\Global Shared Variables.lvlib\\Disk Space Used %"() -> (w843:dbl)  [unwired: 1 in, 1 out]
        n148 = shared-variable ".\\Global Shared Variables.lvlib\\PTP Sync"() -> (w856:bool)  [unwired: 1 in, 1 out]
        n149 = shared-variable ".\\Global Shared Variables.lvlib\\CPU Load Total"() -> (w860:dbl)  [unwired: 1 in, 1 out]
        n150 = local read "MOCCA SO2 Limit"() -> (w802:i32)
        n151 = for {
          tunnel: w854 -> [w1024] mode=indexing
          tunnel: [w1023] -> w851 mode=indexing
          n152 = Boolean To (0,1)(Boolean=w1024) -> (0, 1=w1025:i16)
          n153 = Number To Decimal String(number=w1025, width (-)=i16 1) -> (decimal integer string=w1023:string)
        }
        n154 = Subtract(x=w744, y=w840) -> (x-y=w904:i32)
        n155 = case shown="False" w794 {
          tunnel: [w1017 w1018] -> w891
          tunnel: [w1016 w1019] -> w889
          frame False {
            n156 = local read "10min_so2_avg"() -> (w1017:dbl)
            n157 = local read "8hr_so2_avg 2"() -> (w1016:dbl)
          }
          frame True {
            # "SO2 STEL & TWA simulate"
            n158 = local read "Simulate STEL Conc"() -> (w1018:dbl)
            n159 = local read "Simulate TWA Conc"() -> (w1019:dbl)
          }
        }
        n160 = case shown="True" w870 {
          tunnel: [w1027 w1030] -> w869
          tunnel: [w1026 w1029] -> w868
          tunnel: w866 -> [w1027 _]
          tunnel: w865 -> [w1026 _]
          tunnel: w867 -> [_ w1028]
          frame False {
          }
          frame True {
            w1037 = "_" ("string")
            n161 = Get Date/Time In Seconds() -> (seconds since 1Jan1904=w1038:timestamp)
            n162 = Format Date/Time String(time format string (%c)="%Y%m%d%_%H%M%S", seconds (now)=w1038, UTC format=TRUE) -> (date/time string=w1041:string)
            n163 = Concatenate Strings("TEiSO2-43i" ("string"), w1037, w1041, w1037, w1028, ".txt" ("string")) -> (w1035:string)
            "Default file name" <- w1035
            n164 = Build Path(base path=path "u:/data", name or relative path=w1035) -> (appended path=w1031:path)
            n165 = Open/Create/Replace File(file path (use dialog)=w1031, operation (0:open)=T2."replace or create", access (0:read/write)=enum16{"read/write", "read-only", "write-only"}."write-only") -> (refnum out=w1030:refnum<file>, error out=w1029:errorcluster)  [unwired: 3 in, 1 out]
          }
        }
        n166 = local read "10mins_STEL_limit"() -> (w801:i32)
        n167 = local read "8hr_TWA_limit"() -> (w800:i32)
        n168 = shared-variable ".\\Global Shared Variables.lvlib\\MFM"() -> (w857:dbl)  [unwired: 1 in, 1 out]
        n169 = Number To Decimal String(number=w904) -> (decimal integer string=w903:string)  [unwired: 1 in]
        n170 = Boolean To (0,1)(Boolean=w856) -> (0, 1=w855:i16)
        n171 = Select(t=FALSE, s=w902, f=TRUE) -> (s? t:f=w899:bool)
        "Data Processing" <- w899
        n172 = Number To Decimal String(number=w855) -> (decimal integer string=w782:string)  [unwired: 1 in]
        n173 = Array To Spreadsheet String(delimiter (Tab)=",", array=w851, 3:"%s" ("format string")) -> (spreadsheet string=w842:string)
        n174 = Number To Fractional String(number=w860, precision (6)=i16 2) -> (F-format string=w839:string)  [unwired: 2 in]
        n175 = Number To Fractional String(number=w843, precision (6)=i16 1) -> (F-format string=w838:string)  [unwired: 2 in]
        n176 = To Double Precision Float(number=w800) -> (double precision float=w892:dbl)
        n177 = Number To Fractional String(number=w857, precision (6)=i16 3) -> (F-format string=w774:string)  [unwired: 2 in]
        n178 = Build Array(w803, w802, w801, w800) -> (w799:i32[])
        n179 = To Double Precision Float(number=w801) -> (double precision float=w893:dbl)
        n180 = call <vilib>:"Trim Whitespace.vi"("string"=w842, "location (both)"=w841) -> ("trimmed string"=w763:string)
        n181 = for {
          tunnel: w799 -> [w986] mode=indexing
          tunnel: [w987] -> w805 mode=indexing
          n182 = Number To Decimal String(number=w986) -> (decimal integer string=w987:string)  [unwired: 1 in]
        }
        n183 = local read "MFC 2"() -> (w874:dbl[])
        n184 = local read "MFC 3"() -> (w873:dbl[])
        n185 = local read "Mean Cal\n(default = ON)"() -> (w827:bool)
        n186 = local read "MFC_2 SLPM set value"() -> (w846:dbl)
        n187 = local read "MFC_3 SLPM set value"() -> (w845:dbl)
        n188 = local read "Auto Zeroing"() -> (w813:bool)
        n189 = Greater?(x=w891, y=w893) -> (0:w886:bool)
        n190 = Greater?(x=w889, y=w892) -> (0:w885:bool)
        n191 = Boolean To (0,1)(Boolean=w886) -> (0, 1=w888:i16)
        n192 = local read "ev8 user set time"() -> (w816:i32)
        n193 = Boolean To (0,1)(Boolean=w885) -> (0, 1=w887:i16)
        n194 = call "MFC_Data_Process.vi"("MFC"=w874) -> ("MFC Absolute Pressure"=w773:string, "MFC Temperature"=w772:string, "MFC Volumetric Flow"=w771:string, "MFC Mass Flow"=w770:string, "MFC Set Point"=w769:string)  [unwired: 10 in]
        n195 = call "MFC_Data_Process.vi"("MFC"=w873) -> ("MFC Absolute Pressure"=w768:string, "MFC Temperature"=w767:string, "MFC Volumetric Flow"=w766:string, "MFC Mass Flow"=w765:string, "MFC Set Point"=w764:string)  [unwired: 10 in]
        n196 = local read "ev8 zero interval"() -> (w812:i32)
        n197 = To Unsigned Long Integer(number=w888) -> (unsigned 32bit integer=w884:u32)
        n198 = To Unsigned Long Integer(number=w887) -> (unsigned 32bit integer=w883:u32)
        n199 = Number To Fractional String(number=w891, precision (6)=i16 5) -> (F-format string=w778:string)  [unwired: 2 in]
        n200 = Number To Fractional String(number=w889, precision (6)=i16 5) -> (F-format string=w777:string)  [unwired: 2 in]
        n201 = Array To Spreadsheet String(delimiter (Tab)=",", array=w805, 3:"%s" ("format string")) -> (spreadsheet string=w804:string)
        n202 = Replace Array Subset(array=w882, new element=w934, index=w881) -> (w877:string[])
        "Data Array TCP" <- w877
        n203 = Boolean To (0,1)(Boolean=w813) -> (0, 1=w815:i16)
        n204 = Boolean To (0,1)(Boolean=w784) -> (0, 1=w811:i16)
        n205 = case shown="False" w827 {
          tunnel: [w1020 w1021] -> w824
          frame False {
            n206 = local read "Zero"() -> (w1020:dbl)
          }
          frame True {
            n207 = local read "Mean Cal Offset"() -> (w1021:dbl)
          }
        }
        n208 = call <vilib>:"Trim Whitespace.vi"("string"=w804) -> ("trimmed string"=w753:string)  [unwired: 1 in]
        n209 = To Unsigned Long Integer(number=w815) -> (unsigned 32bit integer=w814:u32)
        n210 = To Unsigned Long Integer(number=w811) -> (unsigned 32bit integer=w810:u32)
        n211 = Index Array(array=w877, index=0) -> (element=w830:string)
        n212 = Concatenate Strings(w914, w920, "\r") -> ()  [unwired: 1 out]
        n213 = Number To Fractional String(number=w845, precision (6)=i16 2) -> (F-format string=w761:string)  [unwired: 2 in]
        n214 = Number To Decimal String(number=w884) -> (decimal integer string=w776:string)  [unwired: 1 in]
        n215 = Number To Decimal String(number=w883) -> (decimal integer string=w775:string)  [unwired: 1 in]
        n216 = Number To Fractional String(number=w846, precision (6)=i16 2) -> (F-format string=w762:string)  [unwired: 2 in]
        n217 = Number To Decimal String(number=w816) -> (decimal integer string=w757:string)  [unwired: 1 in]
        n218 = Number To Decimal String(number=w814, width (-)=i16 1) -> (decimal integer string=w756:string)
        n219 = Number To Decimal String(number=w812) -> (decimal integer string=w755:string)  [unwired: 1 in]
        n220 = Number To Decimal String(number=w810, width (-)=i16 1) -> (decimal integer string=w754:string)
        n221 = Boolean To (0,1)(Boolean=w794) -> (0, 1=w796:i16)
        n222 = local read "Slope"() -> (w823:dbl)
        n223 = Boolean To (0,1)(Boolean=w827) -> (0, 1=w829:i16)
        n224 = local read "Flight Number"() -> (w780:string)
        n225 = To Unsigned Long Integer(number=w796) -> (unsigned 32bit integer=w795:u32)
        n226 = Number To Fractional String(number=w823, precision (6)=i16 2) -> (F-format string=w758:string)  [unwired: 2 in]
        n227 = Number To Decimal String(number=w829, width (-)=i16 1) -> (decimal integer string=w760:string)
        n228 = Number To Fractional String(number=w824, precision (6)=i16 2) -> (F-format string=w759:string)  [unwired: 2 in]
        n229 = Scan From String(format string="%f", input string=w830) -> (output 1=w834:dbl)  [unwired: 3 in, 3 out]
        n230 = Number To Decimal String(number=w795) -> (decimal integer string=w751:string)  [unwired: 1 in]
        n231 = Number To Fractional String(number=w792, precision (6)=i16 2) -> (F-format string=w750:string)  [unwired: 2 in]
        n232 = call "SO2 Calibration Equation.vi"("Input"=w834, "Offset"=w824, "Slope"=w823) -> ("Output"=w820:dbl)  [unwired: 12 in]
        n233 = case shown="True" w784 {
          tunnel: w822 -> [_ w993]
          tunnel: [0 w991] -> w821
          tunnel: w794 -> [_ w996]
          tunnel: w792 -> [_ w995]
          tunnel: w820 -> [_ w994]
          tunnel: [FALSE w992] -> w817
          tunnel: w783 -> [_ w990]
          frame False {
          }
          frame True {
            # "MOCCA SO2 alarm"
            n234 = case shown="True" w990 {
              tunnel: w996 -> [_ w1006]
              tunnel: w995 -> [_ w1005]
              tunnel: w994 -> [_ w1004]
              tunnel: w993 -> [w998 w1003]
              tunnel: [w997 w1001] -> w992
              tunnel: [w998 w1000] -> w991
              frame False {
                n235 = local read "local\ndummy"() -> (w997:bool)
              }
              frame True {
                # "check every 1 second"
                n236 = local read "MOCCA window delay time (sec)"() -> (w1002:i32)
                n237 = Select(t=w1005, s=w1006, f=w1004) -> (s? t:f=w1007:dbl)
                n238 = local read "MOCCA SO2 Limit"() -> (w1008:i32)
                n239 = To Long Integer(number=w1007) -> (32bit integer=w1009:i32)
                n240 = Greater Or Equal?(x=w1009, y=w1008) -> (x >= y?=w999:bool)
                n241 = case shown="True" w999 {
                  tunnel: w1003 -> [_ w1015]
                  tunnel: w1002 -> [_ w1014]
                  tunnel: [FALSE w1013] -> w1001
                  tunnel: [0 w1012] -> w1000
                  frame False {
                  }
                  frame True {
                    n242 = Increment(x=w1015) -> (x+1=w1012:i32)
                    n243 = Greater?(x=w1012, y=w1014) -> (0:w1013:bool)
                  }
                }
                "local\ndummy" <- w1001
              }
            }
          }
        }
        n244 = case shown="True" w783 {
          tunnel: w896 -> [_ w1064]
          tunnel: w820 -> [_ w1061]
          tunnel: w820 -> [_ w1063]
          tunnel: w895 -> [_ w1062]
          tunnel: w836 -> [_ w1055]
          tunnel: w835 -> [w1053 w1060]
          tunnel: w834 -> [_ w1059]
          tunnel: [w1053 w1058] -> w833
          tunnel: w832 -> [w1052 w1057]
          tunnel: [w1052 w1056] -> w831
          frame False {
          }
          frame True {
            # "SO2 monitor every second"
            n245 = local read "Mean Cal\n(default = ON)"() -> (w1054:bool)
            n246 = case shown="True" w1054 {
              tunnel: w1055 -> [_ w1075]
              tunnel: w1060 -> [w1066 w1074]
              tunnel: w1059 -> [_ w1072]
              tunnel: [w1066 w1070] -> w1058
              tunnel: w1057 -> [w1065 w1069]
              tunnel: [w1065 w1068] -> w1056
              frame False {
              }
              frame True {
                w1067 = 5 ("y")
                # "Mean offset calculation - 5 secs after ev8 is turned ON"
                n247 = Equal?(x=w1075, y=TRUE) -> (x = y?=w1077:bool)
                n248 = Increment(x=w1074) -> (x+1=w1076:i32)
                n249 = Select(t=w1076, s=w1077, f=0) -> (s? t:f=w1070:i32)
                n250 = Greater?(x=w1070, y=w1067) -> (0:w1073:bool)
                n251 = case shown="True" w1073 {
                  tunnel: w1072 -> [_ w1084]
                  tunnel: [w1079 w1083] -> w1068
                  tunnel: w1069 -> [w1079 _]
                  tunnel: w1067 -> [_ w1082]
                  frame False {
                  }
                  frame True {
                    n252 = local read "ev8 user set time"() -> (w1080:i32)
                    n253 = Subtract(x=w1080, y=w1082) -> (x-y=w1081:i32)
                    n254 = call <vilib>:"Mean PtByPt.vi"("x"=w1084, "sample length"=w1081) -> ("mean"=w1083:dbl)  [unwired: 2 in, 1 out]
                  }
                }
                "Mean Cal Offset" <- w1068
              }
            }
            n255 = Lossy Enqueue Element(queue=w1064, element=w1061) -> ()  [unwired: 1 in, 4 out]
            n256 = Lossy Enqueue Element(queue=w1062, element=w1063) -> ()  [unwired: 1 in, 4 out]
          }
        }
        n257 = Boolean To (0,1)(Boolean=w817) -> (0, 1=w819:i16)
        n258 = To Unsigned Long Integer(number=w819) -> (unsigned 32bit integer=w818:u32)
        n259 = Number To Decimal String(number=w818, width (-)=i16 1) -> (decimal integer string=w748:string)
        n260 = case shown="True" "Clear Display\nErrors" {
          frame False {
          }
          frame True {
            w1085 = errorcluster {"status"=FALSE, "code"=0, "source"=""} ("UDP Error Out")
            n261 = local write "SEPTIC TCP Error Out"(w1085) -> ()
            n262 = local write "Serial Visa Error"(w1085) -> ()
            n263 = local write "FISH TCP Error Out"(w1085) -> ()
            n264 = local write "UDP_Out_Error"(w1085) -> ()
          }
        }
        n265 = Number To Fractional String(number=w820, precision (6)=i16 5) -> (F-format string=w878:string)  [unwired: 2 in]
        n266 = Replace Array Subset(array=w877, new element=w878, index=0) -> (w876:string[])
        "Data Array UDP" <- w876
        n267 = Array To Spreadsheet String(delimiter (Tab)=",", array=w876, 3:"%s" ("format string")) -> (spreadsheet string=w930:string)
        n268 = call <vilib>:"Trim Whitespace.vi"("string"=w930, "location (both)"=w931) -> ("trimmed string"=w779:string)
        "Data String" <- w779
        n269 = Concatenate Strings(w903, w791, w782, w791, w774, w791, w780, w791, w839, w791, w838, w791, w779, w791, w778, w791, w777, w791, w776, w791, w775, w791, w773, w791, w772, w791, w771, w791, w770, w791, w769, w791, w768, w791, w767, w791, w766, w791, w765, w791, w764, w791, w763, w791, w762, w791, w761, w791, w830, w791, w760, w791, w759, w791, w758, w791, w757, w791, w756, w791, w755, w791, w754, w791, w753, w791, w752, w791, w751, w791, w750, w791, w748) -> (w936:string)
        n270 = Concatenate Strings(w782, w749, "dummy", w749, w780, w749, w774, w749, w778, w749, w777, w749, w776, w749, w775, w749, w773, w749, w772, w749, w771, w749, w770, w749, w769, w749, w768, w749, w767, w749, w766, w749, w765, w749, w764, w749, w763, w749, w762, w749, w761, w749, w760, w749, w759, w749, w758, w749, w757, w749, w756, w749, w755, w749, w754, w749, w753, w749, w752, w749, w751, w749, w750, w749, w748) -> (w747:string)
        n271 = local read "Stop File Write"() -> (w861:bool)
        n272 = call "SO2 TCP Packet_v3.1.vi"("ID"=w746, "Version"=w745, "TCP Packet In"=w747, "utc_time"=w744, "Data Array"=w877) -> ("TCP Binary Packet"=w905:string)  [unwired: 10 in]
        "TCP Binary Packet" <- w905
        n273 = String Length(string=w936) -> (length=w940:i32)
        n274 = Enqueue Element(queue=w907, element=w905, error in (no error)=w906) -> ()  [unwired: 1 in, 3 out]
        n275 = Enqueue Element(queue=w919, element=w905, error in (no error)=w918) -> ()  [unwired: 1 in, 3 out]
        n276 = Number To Decimal String(number=w940, width (-)=i16 3) -> (decimal integer string=w938:string)
        n277 = Concatenate Strings(w746, w745, w937, w938, w937, w936) -> (w862:string)
        "UDP_ASCII_Out" <- w862
        n278 = case shown="False" w861 {
          tunnel: w862 -> [w1047 _]
          tunnel: w869 -> [w1049 w1051]
          tunnel: w868 -> [w1048 w1050]
          tunnel: [w1044 _] -> w864
          tunnel: [w1043 _] -> w863
          frame False {
            n279 = Concatenate Strings(w1047, "\r") -> (w1045:string)
            n280 = Write to Text File(file (use dialog)=w1049, text=w1045, error in=w1048) -> (refnum out=w1044:refnum<file>, error out=w1043:errorcluster)  [unwired: 2 out]
          }
          frame True {
            n281 = Close File(refnum=w1051, error in=w1050) -> ()  [unwired: 2 out]
          }
        }
        n282 = case shown="True" w783 {
          tunnel: w917 -> [_ w1088]
          tunnel: w916 -> [_ w1087]
          tunnel: w862 -> [_ w1086]
          frame False {
          }
          frame True {
            # "Send UDP data once\na second"
            n283 = Enqueue Element(queue=w1088, element=w1086, error in (no error)=w1087) -> ()  [unwired: 1 in, 3 out]
          }
        }
        n284 = local read "stop"() -> (w943:bool)
        n285 = node-c288() -> ()  [unwired: 1 in, 1 out]
      }
      n286 = node-c288() -> (w84:T4)  [unwired: 4 in]
      n287 = node-c288() -> (w86:T4)  [unwired: 4 in]
      n288 = timed-loop {
        tunnel: w90 -> [w428]
        timing: w84 -> [_]
        timing-out: [_] -> w83
        stop <- w429 stop-if-true
        # "10 minutes SO2 Average calculated every second"
        n289 = node-c288() -> ()  [unwired: 1 in, 1 out]
        n290 = Get Queue Status(queue=w428, return elements? (F)=TRUE) -> (elements=w419:dbl[])  [unwired: 1 in, 7 out]
        n291 = for {
          tunnel: w419 -> [w432] mode=indexing
          tunnel: [w436] -> w425
          shift-right: [w435] -> w423
          shift-left: i64 0 -> [w434]
          i -> [w436]
          n292 = To Quad Integer(1:w432) -> (0:w433:i64)
          n293 = Add(x=w434, y=w433) -> (x+y=w435:i64)
        }
        n294 = Increment(x=w425) -> (x+1=w420:i32)
        "q_size" <- w420
        n295 = To Double Precision Float(number=w423) -> (double precision float=w421:dbl)
        n296 = To Double Precision Float(number=w420) -> (double precision float=w422:dbl)
        n297 = Divide(x=w421, y=w422) -> (x/y=→"10min_so2_avg":dbl)
        n298 = local read "stop"() -> (w429:bool)
        n299 = node-c288() -> ()  [unwired: 1 in, 1 out]
      }
      n300 = timed-loop {
        tunnel: w89 -> [w448]
        timing: w86 -> [_]
        timing-out: [_] -> w85
        stop <- w449 stop-if-true
        # "8 hours SO2 Average calculated every second"
        n301 = node-c288() -> ()  [unwired: 1 in, 1 out]
        n302 = Get Queue Status(queue=w448, return elements? (F)=TRUE) -> (elements=w445:dbl[])  [unwired: 1 in, 7 out]
        n303 = for {
          tunnel: w445 -> [w452] mode=indexing
          tunnel: [w456] -> w444
          shift-right: [w455] -> w442
          shift-left: i64 0 -> [w454]
          i -> [w456]
          n304 = To Quad Integer(1:w452) -> (0:w453:i64)
          n305 = Add(x=w454, y=w453) -> (x+y=w455:i64)
        }
        n306 = Increment(x=w444) -> (x+1=w439:i32)
        "q_size 2" <- w439
        n307 = To Double Precision Float(number=w442) -> (double precision float=w440:dbl)
        n308 = To Double Precision Float(number=w439) -> (double precision float=w441:dbl)
        n309 = Divide(x=w440, y=w441) -> (x/y=→"8hr_so2_avg 2":dbl)
        n310 = local read "stop"() -> (w449:bool)
        n311 = node-c288() -> ()  [unwired: 1 in, 1 out]
      }
      n312 = while {
        tunnel: [w603] -> w112
        tunnel: w82 -> [w616]
        tunnel: w81 -> [w615]
        tunnel: [w614] -> w111
        tunnel: w108 -> [w613]
        shift-right: [w611] -> _
        shift-left: 0 -> [w612]
        shift-right: [w609] -> _
        shift-left: u32 0 -> [w610]
        tunnel: w93 -> [w601]
        stop <- "stop" stop-if-true
        w604 = 2
        w606 = string[] ["pmt voltage", "lamp voltage", "lamp int", "internal temp", "react temp", "pres", "flow", "flags"]
        # ">>Monitor command enter as a pair>>"
        # ">>Main commands>>"
        # ">>Monitor Command>>"
        n313 = Array Size(array=w606) -> (size(s)=w607:i32)
        n314 = Divide(x=w607, y=w604) -> (x/y=w605:dbl)
        n315 = for {
          N: w605 -> [_]
          tunnel: w616 -> [w626]
          tunnel: w615 -> [w625]
          tunnel: [w635] -> w603
          shift-right: [w633] -> w611
          shift-left: w612 -> [w634]
          shift-right: [w631] -> w609
          shift-left: w610 -> [w632]
          tunnel: [w630] -> w614
          tunnel: w613 -> [w629]
          tunnel: w606 -> [w622]
          tunnel: "so2" -> [w627]
          tunnel: w604 -> [w623]
          tunnel: w601 -> [w617]
          i -> [w624]
          # "FOR Loop runs according\nto the number of monitor commands"
          # "Assemble command:\nso2\npmt voltage\nlamp voltage\n\netc\netc\n\nso2\nflow\nflags"
          n316 = Multiply(x=w623, y=w624) -> (x*y=w620:i32)
          n317 = Array Subset(array=w622, index=w620, length=w623) -> (w621:string[])
          n318 = Build Array (concatenate)(w627, w621) -> (w628:string[])
          "Data In Array" <- w628
          n319 = node-c288() -> (w619:T4)  [unwired: 4 in]
          n320 = timed-sequence {
            timing: w619 -> [_]
            timing-out: [_] -> w618
            tunnel: w634 -> [w657]
            tunnel: w628 -> [w656]
            tunnel: w626 -> [w655]
            tunnel: w625 -> [w654]
            tunnel: w620 -> [w653]
            tunnel: w629 -> [w648]
            tunnel: [w644] -> w635
            tunnel: [w642] -> w633
            tunnel: w632 -> [w640]
            tunnel: [w639] -> w631
            tunnel: [w638] -> w630
            tunnel: w617 -> [w636]
            n321 = timed-flat-sequence {
              tunnel: w656 -> [w662]
              tunnel: w657 -> [w663]
              tunnel: [w660] -> w652
              tunnel: [w663] -> w651
              tunnel: [w662] -> w650
              tunnel: [w661] -> w649
              tunnel: w655 -> [w660]
              tunnel: [w659] -> w647
              tunnel: w654 -> [w659]
              tunnel: [w658] -> w646
              tunnel: w653 -> [w658]
              tunnel: [w676] -> w645
              tunnel: [w673] -> w643
              tunnel: w652 -> [w668]
              tunnel: w651 -> [w675]
              tunnel: w650 -> [w674]
              tunnel: [w672] -> w641
              tunnel: w649 -> [w672]
              tunnel: [w671] -> w637
              tunnel: w648 -> [w670]
              tunnel: w647 -> [w669]
              tunnel: w646 -> [w667]
              tunnel: w636 -> [w666]
              tunnel: [w738] -> w642
              tunnel: [w739] -> w644
              tunnel: w645 -> [w739]
              tunnel: w643 -> [w738]
              tunnel: w641 -> [w734]
              tunnel: w640 -> [w733]
              tunnel: [w732] -> w639
              tunnel: [w731] -> w638
              tunnel: w637 -> [w731]
              frame #0 {
                n322 = node-c288() -> ()  [unwired: 1 in, 1 out]
                n323 = node-c288() -> ()  [unwired: 1 in, 1 out]
                n324 = Tick Count (ms)() -> (millisecond timer value=w661:u32)
              }
              frame #1 {
                n325 = node-c288() -> ()  [unwired: 1 in, 1 out]
                n326 = while {
                  tunnel: [w690] -> w676
                  tunnel: w674 -> [w688]
                  tunnel: [w686] -> w671
                  tunnel: w670 -> [w685]
                  tunnel: w669 -> [w684]
                  tunnel: w668 -> [w683]
                  tunnel: w667 -> [w682]
                  shift-right: [w687] -> w673
                  shift-left: w675 -> [w689]
                  tunnel: w666 -> [w679]
                  stop <- TRUE stop-if-true
                  # "Receive data is organised as:\nDate Time so2 DATA -1\nDate Time pmt voltage DATA 0\nDate Time lamp voltage DATA 1\nDate Time so2 DATA -1\nDate Time lamp int DATA 2\nDate Time internal temp DATA 3\nDate Time so2 DATA -1\nDate Time react temp DATA 4\nDate Time pres DATA 5\nDate Time so2 DATA -1\nDate Time flow DATA 6\nDate Time flags DATA 7\n\nDate Time Read Error -2"
                  n327 = for {
                    tunnel: w684 -> [w707]
                    tunnel: [w708] -> w690
                    tunnel: w688 -> [w705] mode=indexing
                    tunnel: [w709] -> w686
                    tunnel: w685 -> [w715]
                    tunnel: w683 -> [w710]
                    tunnel: w682 -> [w704]
                    shift-right: [w719] -> w687
                    shift-left: w689 -> [w720]
                    tunnel: w679 -> [w693]
                    i -> [w697]
                    # "Acquire every 330msec for 3 times\nto make 1 second"
                    # "SO2 Acquisition Loop"
                    n328 = call "Wait"("Count(mSec)"=w693) -> ()  [unwired: 1 out]
                    n329 = Concatenate Strings("ID", w705, "\r") -> (w703:string)
                    "Command In" <- w703
                    n330 = call "SO2 Serial Packet Write.vi"("VISA resource name In"=w710, "Data in"=w703, "error in (no error)"=w707) -> ("VISA resource name Out"=w712:refnum<visa-resource-name>, "error out"=w711:errorcluster)  [unwired: 11 in]
                    n331 = call "SO2 Serial Packet Read.vi"("VISA resource In"=w712, "error in"=w711) -> ("VISA resource Out"=w709:refnum<visa-resource-name>, "Data Out"=w700:string, "error out"=w708:errorcluster)  [unwired: 11 in]
                    "RAW DATA" <- w700
                    n332 = Equal?(x=w700, y="Read Error") -> (x = y?=w698:bool)
                    n333 = Get Date/Time In Seconds() -> (seconds since 1Jan1904=w692:timestamp)
                    n334 = case shown="False" w698 {
                      tunnel: [w723 "-2"] -> w713
                      tunnel: w697 -> [w722 _]
                      tunnel: w704 -> [w721 _]
                      frame False {
                        n335 = case shown="0" w722 {
                          tunnel: ["-1" w727 w729] -> w723
                          tunnel: w721 -> [_ w725 w728]
                          frame 0 {
                            # "Make internal flag\n-1 represent so2 data"
                          }
                          frame 2 {
                            # "Make internal flag"
                            n336 = Increment(x=w725) -> (x+1=w726:i32)
                            n337 = Number To Decimal String(number=w726) -> (decimal integer string=w727:string)  [unwired: 1 in]
                          }
                          frame 1, Default {
                            # "Make internal flag"
                            n338 = Number To Decimal String(number=w728) -> (decimal integer string=w729:string)  [unwired: 1 in]
                          }
                        }
                      }
                      frame True {
                      }
                    }
                    n339 = Increment(x=w720) -> (x+1=w716:i32)
                    n340 = Unbundle(w708) -> ("status"=w717:bool)  [unwired: 2 out]
                    n341 = call <vilib>:"Trim Whitespace.vi"("string"=w700) -> ("trimmed string"=w714:string)  [unwired: 1 in]
                    n342 = To Unsigned Long Integer(number=w692) -> (unsigned 32bit integer=w696:u32)
                    n343 = Subtract(x=w696, y=u32 2082844800) -> (x-y=w691:u32)
                    n344 = Select(t=w716, s=w717, f=w720) -> (s? t:f=w719:i32)
                    n345 = call <vilib>:"Space Constant.vi"() -> ("String"=w701:string)
                    n346 = Number To Decimal String(number=w691) -> (decimal integer string=w694:string)  [unwired: 1 in]
                    n347 = Build Array(w694, w701, w714, w701, w713) -> (w702:string[])
                    n348 = Enqueue Element(queue=w715, element=w702) -> ()  [unwired: 2 in, 3 out]
                  }
                  "Number of Send & Read Error\nfrom Acquire Loop" <- w687
                  n349 = call "Wait Until Next Multiple"("Count(mSec)"=u32 1000) -> ()  [unwired: 1 out]
                }
                n350 = node-c288() -> ()  [unwired: 1 in, 1 out]
              }
              frame #2 {
                n351 = node-c288() -> ()  [unwired: 1 in, 1 out]
                n352 = Tick Count (ms)() -> (millisecond timer value=w737:u32)
                n353 = Subtract(x=w737, y=w734) -> (x-y=w736:u32)
                "Acq Time" <- w736
                "Time taken history" <- w736
                n354 = Greater?(x=w736, y=w733) -> (0:w735:bool)
                n355 = Select(t=w736, s=w735, f=w733) -> (s? t:f=w732:u32)
                "Max Acq Time diff" <- w732
                n356 = node-c288() -> ()  [unwired: 1 in, 1 out]
              }
            }
          }
          n357 = node-c288(w618) -> ()  [unwired: 1 out]
        }
      }
      n358 = node-c288(w85) -> ()  [unwired: 1 out]
      n359 = node-c288(w83) -> ()  [unwired: 1 out]
      n360 = while {
        stop <- FALSE stop-if-true
        # "CAL MFC 3 status & control"
        n361 = Wait (ms)(milliseconds to wait=u32 1000) -> ()  [unwired: 1 out]
        n362 = call-poly "VISA Configure Serial Port"("VISA resource name"="VISA resource name 2", "timeout (10sec)"="timeout (10sec) 2", "termination char\n(0xA = '\\n' = LF)"=u8 13 ("termination char\n(0xA = '\\n' = LF)"), "Enable Termination\nChar (T)"=TRUE ("Enable Termination\nChar (T)"), "baud rate (9600)"=u32 19200) -> ("VISA resource name out"=w360:refnum<visa-resource-name>, "error out"=w356:errorcluster)  [unwired: 9 in]
        n363 = case shown="No Error" w356 {
          selector: w356 -> [w367 w417]
          tunnel: w360 -> [w368 w418]
          tunnel: [w366 w418] -> w359
          tunnel: [w365 w417] -> w358
          frame No Error {
            n364 = node-c288() -> (w363:T4)  [unwired: 4 in]
            n365 = timed-loop {
              tunnel: w368 -> [w391]
              tunnel: w367 -> [w389]
              tunnel: [w382] -> w366
              tunnel: [w377] -> w365
              shift-right: [w378] -> _
              shift-left: FALSE -> [w381]
              timing: w363 -> [_]
              timing-out: [_] -> w362
              shift-right: [w369] -> _
              shift-left: 0.0 -> [w371]
              stop <- w377 stop-if-true
              n366 = node-c288() -> ()  [unwired: 1 in, 1 out]
              n367 = local read "MFC_3 SLPM set value"() -> (w369:dbl)
              n368 = Not Equal?(x=w369, y=w371) -> (x != y?=w370:bool)
              n369 = case shown="True" w370 {
                tunnel: w391 -> [w399 w414]
                tunnel: [w399 w414] -> w390
                tunnel: w389 -> [w398 w413]
                tunnel: [w398 w413] -> w388
                tunnel: "A" -> [w402 w406]
                tunnel: [w400 w403] -> w386
                frame False {
                  n370 = Concatenate Strings(w402, "\r") -> (w400:string)
                }
                frame True {
                  n371 = Multiply(x="MFC_3 SLPM set value", y=u32 64000) -> (x*y=w410:dbl)
                  n372 = Divide(x=w410, y=u32 5) -> (x/y=w408:dbl)
                  n373 = To Unsigned Long Integer(number=w408) -> (unsigned 32bit integer=w407:u32)
                  n374 = Number To Decimal String(number=w407) -> (decimal integer string=w405:string)  [unwired: 1 in]
                  n375 = Concatenate Strings(w406, w405, "\r") -> (w403:string)
                }
              }
              n376 = VISA Flush I/O Buffer(VISA resource name=w390, error in (no error)=w388) -> (VISA resource name out=w393:refnum<visa-resource-name>, error out=w392:errorcluster)  [unwired: 1 in]
              n377 = Select(t=FALSE, s=w381, f=TRUE) -> (s? t:f=w378:bool)
              "status" <- w378
              n378 = VISA Write(VISA resource name=w393, write buffer=w386, error in (no error)=w392) -> (VISA resource name out=w385:refnum<visa-resource-name>, error out=w384:errorcluster)  [unwired: 1 out]
              n379 = VISA Flush I/O Buffer(VISA resource name=w385, error in (no error)=w384) -> (VISA resource name out=w395:refnum<visa-resource-name>, error out=w394:errorcluster)  [unwired: 1 in]
              n380 = VISA Read(VISA resource name=w395, byte count=u32 50, error in (no error)=w394) -> (VISA resource name out=w382:refnum<visa-resource-name>, read buffer=w376:string, error out=w377:errorcluster)  [unwired: 1 out]
              "Value Read 3" <- w376
              n381 = call <vilib>:"Space Constant.vi"() -> ("String"=w375:string)
              n382 = Spreadsheet String To Array(delimiter (Tab)=w375, format string="%f", spreadsheet string=w376, array type (2D Dbl)=dbl[] []) -> (array=→"MFC 3":dbl[])
              n383 = node-c288() -> ()  [unwired: 1 in, 1 out]
            }
            n384 = node-c288(w362) -> ()  [unwired: 1 out]
          }
          frame Error {
          }
        }
        n385 = VISA Close(VISA resource name=w359, error in (no error)=w358) -> (error out=→"error out 3":errorcluster)
      }
      n386 = while {
        stop <- FALSE stop-if-true
        # "CAL MFC 2 status & control"
        n387 = Wait (ms)(milliseconds to wait=u32 1000) -> ()  [unwired: 1 out]
        n388 = call-poly "VISA Configure Serial Port"("VISA resource name"="VISA resource name 3", "timeout (10sec)"="timeout (10sec) 3", "termination char\n(0xA = '\\n' = LF)"=u8 13 ("termination char\n(0xA = '\\n' = LF)"), "Enable Termination\nChar (T)"=TRUE ("Enable Termination\nChar (T)"), "baud rate (9600)"=u32 19200) -> ("VISA resource name out"=w290:refnum<visa-resource-name>, "error out"=w286:errorcluster)  [unwired: 9 in]
        n389 = case shown="No Error" w286 {
          selector: w286 -> [w297 w347]
          tunnel: w290 -> [w298 w348]
          tunnel: [w296 w348] -> w289
          tunnel: [w295 w347] -> w288
          frame No Error {
            n390 = node-c288() -> (w293:T4)  [unwired: 4 in]
            n391 = timed-loop {
              tunnel: w298 -> [w321]
              tunnel: w297 -> [w319]
              tunnel: [w312] -> w296
              tunnel: [w307] -> w295
              shift-right: [w308] -> _
              shift-left: FALSE -> [w311]
              timing: w293 -> [_]
              timing-out: [_] -> w292
              shift-right: [w299] -> _
              shift-left: 0.0 -> [w301]
              stop <- w307 stop-if-true
              n392 = node-c288() -> ()  [unwired: 1 in, 1 out]
              n393 = local read "MFC_2 SLPM set value"() -> (w299:dbl)
              n394 = Not Equal?(x=w299, y=w301) -> (x != y?=w300:bool)
              n395 = case shown="True" w300 {
                tunnel: w321 -> [w329 w344]
                tunnel: [w329 w344] -> w320
                tunnel: w319 -> [w328 w343]
                tunnel: [w328 w343] -> w318
                tunnel: "A" -> [w332 w336]
                tunnel: [w330 w333] -> w316
                frame False {
                  n396 = Concatenate Strings(w332, "\r") -> (w330:string)
                }
                frame True {
                  n397 = Multiply(x="MFC_2 SLPM set value", y=u32 64000) -> (x*y=w340:dbl)
                  n398 = Divide(x=w340, y=u32 5) -> (x/y=w338:dbl)
                  n399 = To Unsigned Long Integer(number=w338) -> (unsigned 32bit integer=w337:u32)
                  n400 = Number To Decimal String(number=w337) -> (decimal integer string=w335:string)  [unwired: 1 in]
                  n401 = Concatenate Strings(w336, w335, "\r") -> (w333:string)
                }
              }
              n402 = Select(t=FALSE, s=w311, f=TRUE) -> (s? t:f=w308:bool)
              "status 2" <- w308
              n403 = VISA Flush I/O Buffer(VISA resource name=w320, error in (no error)=w318) -> (VISA resource name out=w323:refnum<visa-resource-name>, error out=w322:errorcluster)  [unwired: 1 in]
              n404 = VISA Write(VISA resource name=w323, write buffer=w316, error in (no error)=w322) -> (VISA resource name out=w315:refnum<visa-resource-name>, error out=w314:errorcluster)  [unwired: 1 out]
              n405 = VISA Flush I/O Buffer(VISA resource name=w315, error in (no error)=w314) -> (VISA resource name out=w325:refnum<visa-resource-name>, error out=w324:errorcluster)  [unwired: 1 in]
              n406 = VISA Read(VISA resource name=w325, byte count=u32 50, error in (no error)=w324) -> (VISA resource name out=w312:refnum<visa-resource-name>, read buffer=w306:string, error out=w307:errorcluster)  [unwired: 1 out]
              "Value Read 2" <- w306
              n407 = call <vilib>:"Space Constant.vi"() -> ("String"=w305:string)
              n408 = Spreadsheet String To Array(delimiter (Tab)=w305, format string="%f", spreadsheet string=w306, array type (2D Dbl)=dbl[] []) -> (array=→"MFC 2":dbl[])
              n409 = node-c288() -> ()  [unwired: 1 in, 1 out]
            }
            n410 = node-c288(w292) -> ()  [unwired: 1 out]
          }
          frame Error {
          }
        }
        n411 = VISA Close(VISA resource name=w289, error in (no error)=w288) -> (error out=→"error out 2":errorcluster)
      }
      n412 = node-c288(w109) -> ()  [unwired: 1 out]
      n413 = while {
        stop <- FALSE stop-if-true
        n414 = node-c288() -> (w119:T4)  [unwired: 4 in]
        n415 = Create Network Stream Reader Endpoint(7:10 ("reader buffer size"), 9:T3 {"Message"="", "Message Data"=variant} ("Message Cluster"), 11:"/command/reader/SO2" ("reader url")) -> (0:w125:errorcluster, 3:w126:refnum<k21>)  [unwired: 4 in]
        n416 = timed-loop "Host->Target Command Reader" {
          shift-right: [w136] -> w123
          shift-left: w125 -> [w139]
          shift-right: [w137] -> w122
          shift-left: w126 -> [w138]
          tunnel: [TRUE] -> _
          timing: w119 -> [_]
          timing-out: [_] -> w118
          stop <- w130 stop-if-true
          # "Receive Commands from Host VI"
          n417 = node-c288() -> ()  [unwired: 1 in, 1 out]
          n418 = shared-variable-read(w138, w139) -> (w137:refnum<k21>, w132:errorcluster, w134:bool, w135:T3)  [unwired: 1 in]
          n419 = Or(x=w134, y=w132) -> (x .or. y?=w133:bool)
          n420 = case shown="False" w133 {
            selector: w133 -> [_ w275]
            tunnel: w132 -> [w147 w276]
            tunnel: [w146 w276] -> w136
            tunnel: w135 -> [w144 _]
            tunnel: [w145 w275] -> w130
            frame False {
              n421 = Unbundle By Name(w144) -> ("Message"=w143:string, "Message Data"=w142:variant)
              n422 = case shown="\"V6\"" w143 {
                tunnel: w147 -> [w149 w154 w159 w164 w169 w174 w179 w184 w189 w194 w199 w204 w209 w214 w219 w224 w229 w234 w239 w244 w249 w254 w259 w263 w268 w273]
                tunnel: [w149 w153 w158 w163 w168 w173 w178 w183 w188 w193 w198 w203 w208 w213 w218 w223 w228 w233 w238 w243 w248 w253 w258 w261 w266 w271] -> w146
                tunnel: w142 -> [_ w152 w157 w162 w167 w172 w177 w182 w187 w192 w197 w202 w207 w212 w217 w222 w227 w232 w237 w242 w247 w252 w257 w264 w269 w274]
                tunnel: [TRUE _ _ _ _ _ _ _ _ _ _ _ _ _ _ _ _ _ _ _ _ _ _ _ _ _] -> w145
                frame "Stop", Default {
                }
                frame "V9" {
                  n423 = Variant To Data(error in=w154, type=FALSE, Variant=w152) -> (data=w150:bool, error out=w153:errorcluster)
                  "V9" <- w150
                  n424 = shared-variable "NI-cRIO9022-019C2C95\\Mod6\\DO7"(w150) -> ()  [unwired: 1 in, 1 out]
                }
                frame "MFC_2" {
                  n425 = Variant To Data(error in=w159, type=0.0, Variant=w157) -> (data=w155:dbl, error out=w158:errorcluster)
                  n426 = local write "MFC_2 SLPM set value"(w155) -> ()
                }
                frame "cal_gas_cylin_conc" {
                  n427 = Variant To Data(error in=w164, type=0.0, Variant=w162) -> (data=→"cal gas cylinder conc":dbl, error out=w163:errorcluster)
                }
                frame "sim_MOCCA_conc" {
                  n428 = Variant To Data(error in=w169, type=0.0, Variant=w167) -> (data=→"Simulate MOCCA Conc":dbl, error out=w168:errorcluster)
                }
                frame "Auto_zero" {
                  n429 = Variant To Data(error in=w174, type=FALSE, Variant=w172) -> (data=→"Auto Zeroing":bool, error out=w173:errorcluster)
                }
                frame "zeroing_interval" {
                  n430 = Variant To Data(error in=w179, type=0, Variant=w177) -> (data=→"ev8 zero interval":i32, error out=w178:errorcluster)
                }
                frame "MOCCA_window_delay_time" {
                  n431 = Variant To Data(error in=w184, type=0, Variant=w182) -> (data=→"MOCCA window delay time (sec)":i32, error out=w183:errorcluster)
                }
                frame "MOCCA_limit" {
                  n432 = Variant To Data(error in=w189, type=0, Variant=w187) -> (data=→"MOCCA SO2 Limit":i32, error out=w188:errorcluster)
                }
                frame "eV8_user_set_time" {
                  n433 = Variant To Data(error in=w194, type=0, Variant=w192) -> (data=→"ev8 user set time":i32, error out=w193:errorcluster)
                }
                frame "MFC_3" {
                  n434 = Variant To Data(error in=w199, type=0.0, Variant=w197) -> (data=w195:dbl, error out=w198:errorcluster)
                  n435 = local write "MFC_3 SLPM set value"(w195) -> ()
                }
                frame "Simulate STEL Conc" {
                  n436 = Variant To Data(error in=w204, type=0.0, Variant=w202) -> (data=→"Simulate STEL Conc":dbl, error out=w203:errorcluster)
                }
                frame "Simulate TWA Conc" {
                  n437 = Variant To Data(error in=w209, type=0.0, Variant=w207) -> (data=→"Simulate TWA Conc":dbl, error out=w208:errorcluster)
                }
                frame "Offset" {
                  n438 = Variant To Data(error in=w214, type=0.0, Variant=w212) -> (data=→"Zero":dbl, error out=w213:errorcluster)
                }
                frame "10mins STEL Limit" {
                  n439 = Variant To Data(error in=w219, type=0, Variant=w217) -> (data=→"10mins_STEL_limit":i32, error out=w218:errorcluster)
                }
                frame "UDP Time Offset" {
                  n440 = Variant To Data(error in=w224, type=0, Variant=w222) -> (data=→"UDP Time Stamp Offset":i32, error out=w223:errorcluster)
                }
                frame "8hr TWA Limit" {
                  n441 = Variant To Data(error in=w229, type=0, Variant=w227) -> (data=→"8hr_TWA_limit":i32, error out=w228:errorcluster)
                }
                frame "Slope" {
                  n442 = Variant To Data(error in=w234, type=0.0, Variant=w232) -> (data=→"Slope":dbl, error out=w233:errorcluster)
                }
                frame "V8" {
                  n443 = Variant To Data(error in=w239, type=FALSE, Variant=w237) -> (data=w235:bool, error out=w238:errorcluster)
                  "V8" <- w235
                  n444 = shared-variable "NI-cRIO9022-019C2C95\\Mod6\\DO6"(w235) -> ()  [unwired: 1 in, 1 out]
                }
                frame "Stop File Write" {
                  n445 = Variant To Data(error in=w244, type=FALSE, Variant=w242) -> (data=→"Stop File Write":bool, error out=w243:errorcluster)
                }
                frame "SO2_MOCCA_Alarm" {
                  n446 = Variant To Data(error in=w249, type=FALSE, Variant=w247) -> (data=→"SO2 Inflight MOCCA Alarm\n(default = OFF)":bool, error out=w248:errorcluster)
                }
                frame "Flight Number" {
                  n447 = Variant To Data(error in=w254, type="", Variant=w252) -> (data=→"Flight Number":string, error out=w253:errorcluster)
                }
                frame "V6" {
                  n448 = Variant To Data(error in=w259, type=FALSE, Variant=w257) -> (data=w255:bool, error out=w258:errorcluster)
                  "V6" <- w255
                  n449 = shared-variable "NI-cRIO9022-019C2C95\\Mod6\\DO4"(w255) -> ()  [unwired: 1 in, 1 out]
                }
                frame "Simulate Conc" {
                  n450 = Variant To Data(error in=w263, type=FALSE, Variant=w264) -> (data=→"Simulate\nconc":bool, error out=w261:errorcluster)
                }
                frame "calcon_save" {
                  n451 = Variant To Data(error in=w268, type=FALSE, Variant=w269) -> (data=→"calcon save to file":bool, error out=w266:errorcluster)
                }
                frame "mean_cal_status" {
                  n452 = Variant To Data(error in=w273, type=FALSE, Variant=w274) -> (data=→"Mean Cal\n(default = ON)":bool, error out=w271:errorcluster)
                }
              }
            }
            frame True {
            }
          }
          n453 = node-c288() -> ()  [unwired: 1 in, 1 out]
        }
        n454 = node-c288(w118) -> ()  [unwired: 1 out]
        n455 = Destroy Stream Endpoint(8:w123, 11:w122) -> (0:→"error out 4":errorcluster)
        n456 = Wait (ms)(milliseconds to wait=u32 1000) -> ()  [unwired: 1 out]
      }
      n457 = while {
        tunnel: w96 -> [w502]
        stop <- w503 stop-if-true
        # "UDP Broadcast loop"
        # "Broadcast UDP SO2 Data"
        n458 = node-c288() -> (w505:T4)  [unwired: 4 in]
        n459 = String To IP(1:"239.1.4.6" ("name")) -> (0:w507:u32)
        n460 = call-poly <vilib>:"UDP Multicast Open.vi"("time-to-live (1)"=u16 5, "port"=u16 10001) -> ("error out"=w515:errorcluster, "connection ID"=w516:refnum<k16>)  [unwired: 8 in]
        n461 = timed-loop {
          tunnel: w516 -> [w536]
          tunnel: w515 -> [w535]
          tunnel: [w522] -> w511
          shift-right: [w525] -> _
          shift-left: FALSE -> [w528]
          tunnel: [w520] -> w509
          tunnel: w507 -> [w524]
          tunnel: u16 50001 ("port or service name") -> [w523]
          timing: w505 -> [_]
          timing-out: [_] -> w504
          tunnel: [w518] -> w503
          tunnel: w502 -> [w517]
          stop <- w519 stop-if-true
          n462 = node-c288() -> ()  [unwired: 1 in, 1 out]
          n463 = local read "Flight Number"() -> (w531:string)
          n464 = Select(t=FALSE, s=w528, f=TRUE) -> (s? t:f=w525:bool)
          "UDP packet \nstatus" <- w525
          n465 = feedback-in #2(w531) -> ()
          n466 = feedback #2() -> (w530:string)  [unwired: 1 in]
          n467 = Not Equal?(x=w531, y=w530) -> (x != y?=w529:bool)
          n468 = flat-sequence {
            tunnel: w524 -> [w544]
            tunnel: w535 -> [w545]
            tunnel: w536 -> [w546]
            tunnel: [w546] -> w534
            tunnel: [w545] -> w533
            tunnel: [w544] -> w532
            tunnel: w529 -> [w543]
            tunnel: w523 -> [w556]
            tunnel: w534 -> [w555]
            tunnel: w533 -> [w554]
            tunnel: w532 -> [w553]
            tunnel: [w552] -> w522
            tunnel: [w551] -> w520
            tunnel: w517 -> [w550]
            frame #0 {
              n469 = feedback #3(u32 0) -> (w540:u32)
              n470 = case shown="True" w543 {
                tunnel: w540 -> [w547 _]
                tunnel: [w547 u32 0] -> w539
                frame False {
                }
                frame True {
                }
              }
              "UDP_Pack_num" <- w539
              n471 = Increment(x=w539) -> (x+1=w541:u32)
              n472 = feedback-in #3(w541) -> ()
            }
            frame #1 {
              n473 = Dequeue Element(queue=w550) -> (element=w549:string)  [unwired: 2 in, 3 out]
              n474 = UDP Write(address=w553, port or service name=w556, connection ID=w555, data in=w549, 8:w554) -> (error out=w551:errorcluster, 3:w552:refnum<k16>)  [unwired: 1 in]
            }
          }
          n475 = local read "stop"() -> (w518:bool)
          n476 = Unbundle(w520) -> ("status"=w521:bool)  [unwired: 2 out]
          n477 = node-c288() -> ()  [unwired: 1 in, 1 out]
          n478 = Compound Arithmetic op=OR(w521, w518) -> (w519:bool)
        }
        n479 = node-c288(w504) -> ()  [unwired: 1 out]
        n480 = UDP Close(connection ID=w511, 8:w509) -> (error out=→"UDP_Out_Error":errorcluster)  [unwired: 1 out]
        n481 = Wait (ms)(milliseconds to wait=u32 1000) -> ()  [unwired: 1 out]
      }
      n482 = while {
        stop <- FALSE stop-if-true
        # "Emergency shutdown on the valves when connection to the client drops"
        n483 = shared-variable ".\\Global Shared Variables.lvlib\\Disconnect_WatchDog"() -> (w113:bool)  [unwired: 1 in, 1 out]
        n484 = Wait (ms)(milliseconds to wait=u32 1000) -> ()  [unwired: 1 out]
        n485 = case shown="True" w113 {
          frame False {
          }
          frame True {
            w116 = FALSE
            n486 = shared-variable "NI-cRIO9022-019C2C95\\Mod6\\DO4"(w116) -> ()  [unwired: 1 in, 1 out]
            n487 = shared-variable "NI-cRIO9022-019C2C95\\Mod6\\DO7"(w116) -> ()  [unwired: 1 in, 1 out]
            n488 = shared-variable "NI-cRIO9022-019C2C95\\Mod6\\DO6"(w116) -> ()  [unwired: 1 in, 1 out]
            n489 = local write "MFC_2 SLPM set value"(0.0 ("MFC_2 SLPM set value")) -> ()
          }
        }
      }
      n490 = while {
        tunnel: w94 -> [w461]
        tunnel: w95 -> [w460]
        stop <- w464 stop-if-true
        # "TCP Loop writing to SEPTIC Tank"
        n491 = TCP Open Connection(address="192.168.101.108", remote port or service name=u16 3502) -> (connection ID=w467:refnum<k5>, error out=w462:errorcluster)  [unwired: 3 in]
        n492 = case shown="No Error" w462 {
          selector: w462 -> [w472 w499]
          tunnel: w467 -> [w477 w500]
          tunnel: [w476 w500] -> w466
          tunnel: [w475 w499] -> w465
          tunnel: [w474 w498] -> w464
          tunnel: w460 -> [w471 _]
          tunnel: w461 -> [w470 _]
          frame No Error {
            n493 = node-c288() -> (w479:T4)  [unwired: 4 in]
            n494 = timed-loop {
              tunnel: w477 -> [w493]
              tunnel: w472 -> [w492]
              tunnel: [w491] -> w476
              tunnel: [w490] -> w475
              tunnel: [w480] -> w474
              shift-right: [w484] -> _
              shift-left: FALSE -> [w487]
              timing: w479 -> [_]
              timing-out: [_] -> w478
              tunnel: w471 -> [w483]
              tunnel: w470 -> [w482]
              stop <- w488 stop-if-true
              n495 = node-c288() -> ()  [unwired: 1 in, 1 out]
              n496 = Dequeue Element(queue=w483, error in (no error)=w482) -> (element=w481:string)  [unwired: 1 in, 3 out]
              n497 = Select(t=FALSE, s=w487, f=TRUE) -> (s? t:f=w484:bool)
              "TCP packet\nSend to SEPTIC" <- w484
              n498 = TCP Write(connection ID=w493, data in=w481, error in (no error)=w492) -> (connection ID out=w491:refnum<k5>, error out=w490:errorcluster)  [unwired: 1 in, 1 out]
              n499 = local read "stop"() -> (w480:bool)
              n500 = Unbundle(w490) -> ("status"=w489:bool)  [unwired: 2 out]
              n501 = node-c288() -> ()  [unwired: 1 in, 1 out]
              n502 = Compound Arithmetic op=OR(w489, w480) -> (w488:bool)
            }
            n503 = node-c288(w478) -> ()  [unwired: 1 out]
          }
          frame Error {
            n504 = local read "stop"() -> (w498:bool)
          }
        }
        n505 = TCP Close Connection(connection ID=w466, error in (no error)=w465) -> (error out=→"SEPTIC TCP Error Out":errorcluster)  [unwired: 1 in, 1 out]
        n506 = Wait (ms)(milliseconds to wait=u32 1000) -> ()  [unwired: 1 out]
      }
      n507 = while {
        tunnel: w100 -> [w561]
        tunnel: w99 -> [w560]
        stop <- w564 stop-if-true
        # "TCP Loop writing to FISH Tank"
        n508 = TCP Open Connection(address="192.168.101.110", remote port or service name=u16 3502) -> (connection ID=w567:refnum<k5>, error out=w562:errorcluster)  [unwired: 3 in]
        n509 = case shown="No Error" w562 {
          selector: w562 -> [w572 w599]
          tunnel: w567 -> [w577 w600]
          tunnel: [w576 w600] -> w566
          tunnel: [w575 w599] -> w565
          tunnel: [w574 w598] -> w564
          tunnel: w561 -> [w571 _]
          tunnel: w560 -> [w570 _]
          frame No Error {
            n510 = node-c288() -> (w579:T4)  [unwired: 4 in]
            n511 = timed-loop {
              tunnel: w577 -> [w593]
              tunnel: w572 -> [w592]
              tunnel: [w591] -> w576
              tunnel: [w590] -> w575
              tunnel: [w587] -> w574
              shift-right: [w583] -> _
              shift-left: FALSE -> [w586]
              timing: w579 -> [_]
              timing-out: [_] -> w578
              tunnel: w571 -> [w582]
              tunnel: w570 -> [w581]
              stop <- w588 stop-if-true
              n512 = node-c288() -> ()  [unwired: 1 in, 1 out]
              n513 = Dequeue Element(queue=w582, error in (no error)=w581) -> (element=w580:string)  [unwired: 1 in, 3 out]
              n514 = Select(t=FALSE, s=w586, f=TRUE) -> (s? t:f=w583:bool)
              "TCP packet\nSend to FISH" <- w583
              n515 = TCP Write(connection ID=w593, data in=w580, error in (no error)=w592) -> (connection ID out=w591:refnum<k5>, error out=w590:errorcluster)  [unwired: 1 in, 1 out]
              n516 = local read "stop"() -> (w587:bool)
              n517 = Unbundle(w590) -> ("status"=w589:bool)  [unwired: 2 out]
              n518 = node-c288() -> ()  [unwired: 1 in, 1 out]
              n519 = Compound Arithmetic op=OR(w589, w587) -> (w588:bool)
            }
            n520 = node-c288(w578) -> ()  [unwired: 1 out]
          }
          frame Error {
            n521 = local read "stop"() -> (w598:bool)
          }
        }
        n522 = TCP Close Connection(connection ID=w566, error in (no error)=w565) -> (error out=→"FISH TCP Error Out":errorcluster)  [unwired: 1 in, 1 out]
        n523 = Wait (ms)(milliseconds to wait=u32 1000) -> ()  [unwired: 1 out]
      }
    }
    frame Error {
    }
  }
  n524 = VISA Close(VISA resource name=w36, error in (no error)=w35) -> (error out=→"Serial Visa Error":errorcluster)
